vi "PVCamApp.vi"() -> ()   [LabVIEW 2018]
uses:
  D:/SVN/PM/sdk/AppSamples/LabVIEWSamples/trunk/Release/2018/Dependencies/PVCamNET.dll
  Dependencies/PVCamNET.dll
  SubVis/PVCamGlobalVariables.vi
panel:
  out "Name":string
  in  "Bayer pattern":string(combo)
  in  "Camera Control":enum32{"Basic", "Advanced", "Disk streaming"}(tab)
  out "Disk queue size":dbl
  out "Buffer Index":dbl
  in  "Scrollbar":i32(c297)
  in  "Exposure Time":dbl
  in  "Binning":string(combo)
  in  "X":u16
  in  "Width":u16
  in  "Y":u16
  in  "Height":u16
  in  "Full CCD":bool
  in  "Single Capture":bool
  in  "Live start":bool
  in  "Live stop":bool
  in  "Live status":bool
  in  "Get ROI":bool
  in  "Save Image to TIFF":bool
  out "Capturing":bool
  in  "Exposure Resolution":string(combo)
  out "8 Bit Histogram":i32[](graph)
  in  "Histogram On/Off":bool
  out "?":string
  out "Image saving path":string
  in  "Color (Off/On)":bool
  in  "Post-processing function value":dbl
  in  "Post-processing function":string(combo)
  in  "Readout ports and speeds":string(combo)
  in  "Gain":string(combo)
  in  "Sensor clearing mode":string(combo)
  in  "Clear Cycles":dbl
  in  "Trigger Out Behavior":string(combo)
  in  "Trigger In Behavior":string(combo)
  out "Stream Saving":bool
  in  "Disk streaming On/Off":bool
  in  "Format (0 for RAW[mono only] and 1 for TIFF[mono/color])":u8 max=1 step=1
  out "Disk stream saving path":string
  in  "Image saving path":path
  out "LabVIEW app version":string
  out "PVCamNET version":string
  out "Trigger Mode":i32
  out "Exposure":u32
  out "YBinning":u16
  out "XBinning":u16
  out "CC Min":u32
  out "CC Max":u32
  out "Exp. out":i32
  out "Clearing modes":i32
  out "Full CCD Y":i32
  out "Full CCD Height":i32
  out "Full CCD Width":i32
  out "Full CCD X":i32
  out "Y Binning":u32
  out "X Binning":u32
  in  "Init":bool
  in  "Camera status":bool
  in  "Close Camera":bool
  in  "Open Camera":bool
  in  "Select Camera":string(combo)
  in  "Uninit":bool
  in  "PVCam indicator":bool
  out "PVCam version":string
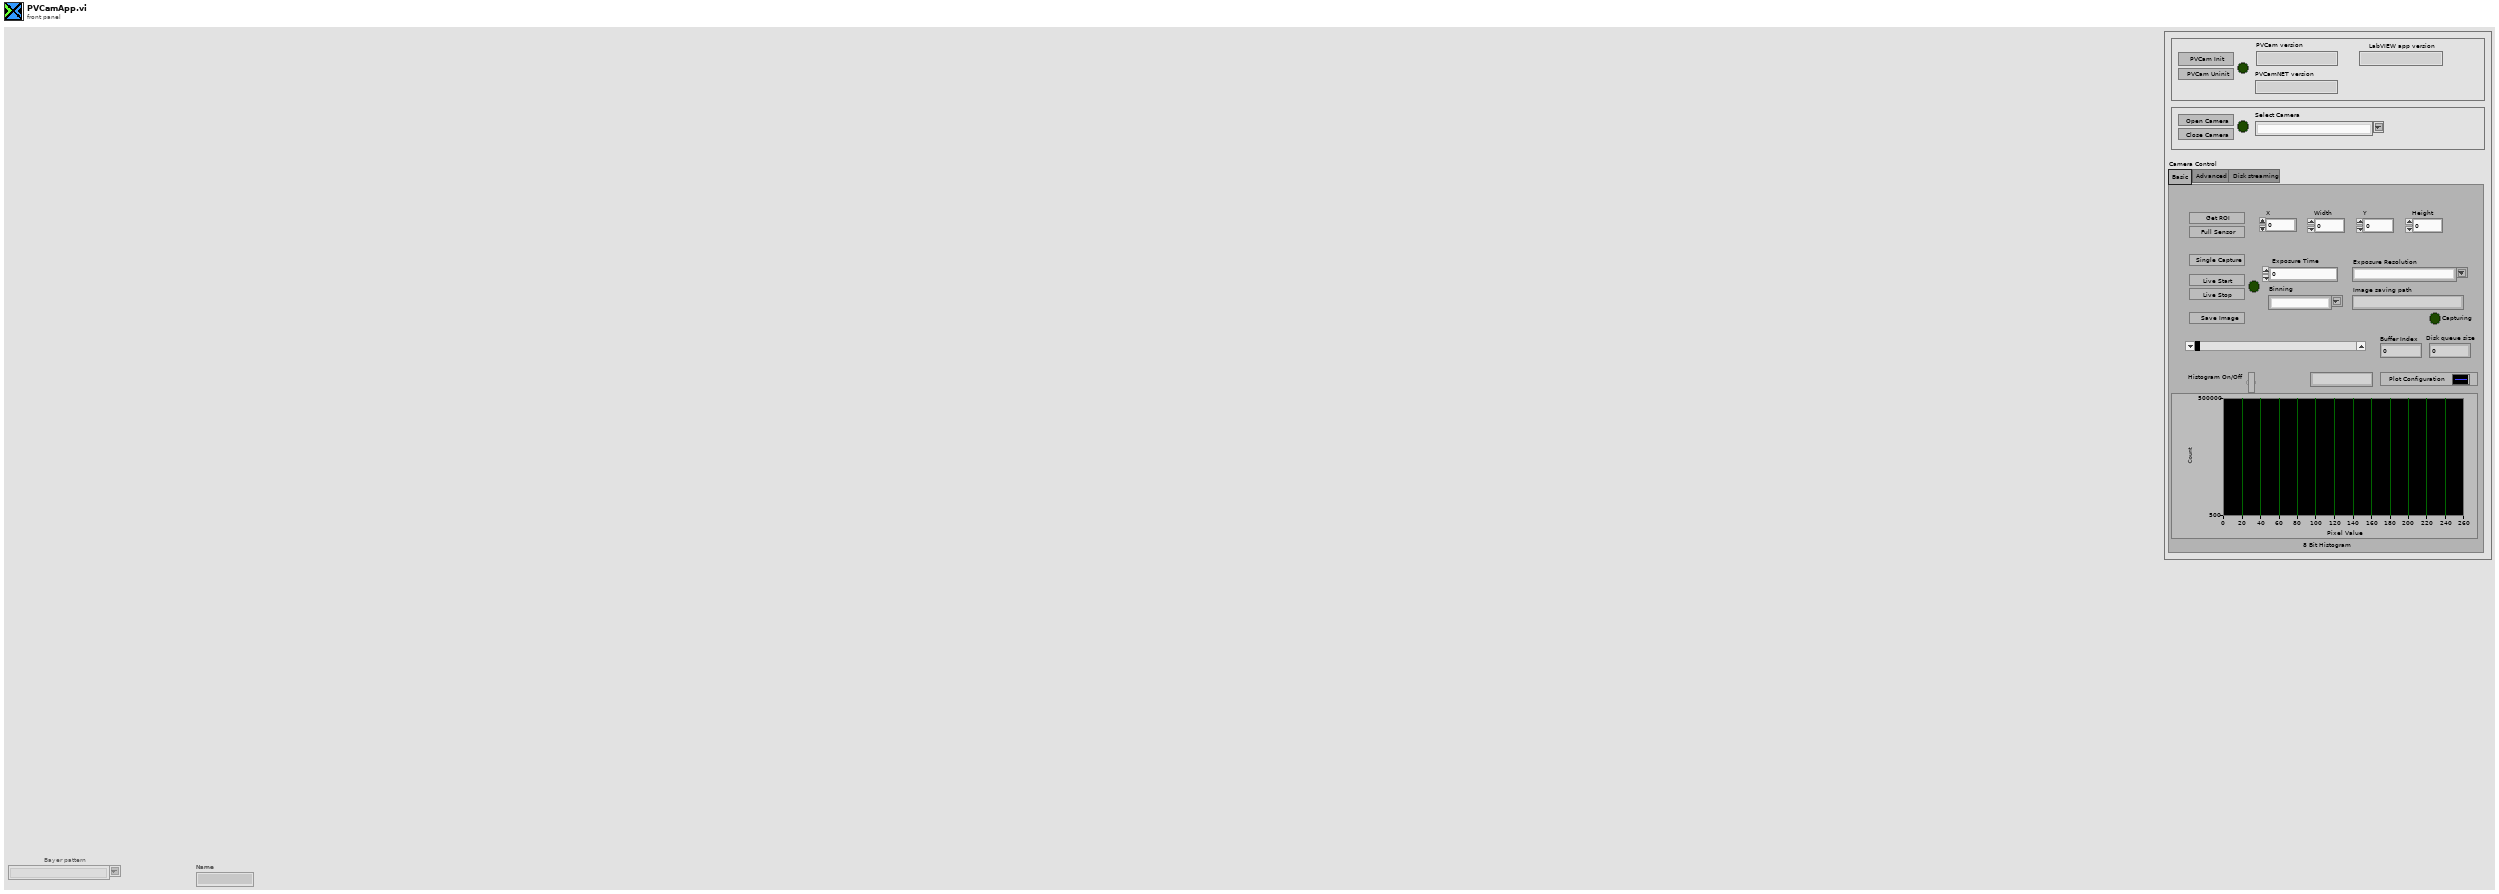
[diagram p1: front panel]
types:
  T1 = cluster{"Buffer Index":refnum<vi>, "Disk queue size":refnum<vi>, "Scrollbar":refnum<vi>}
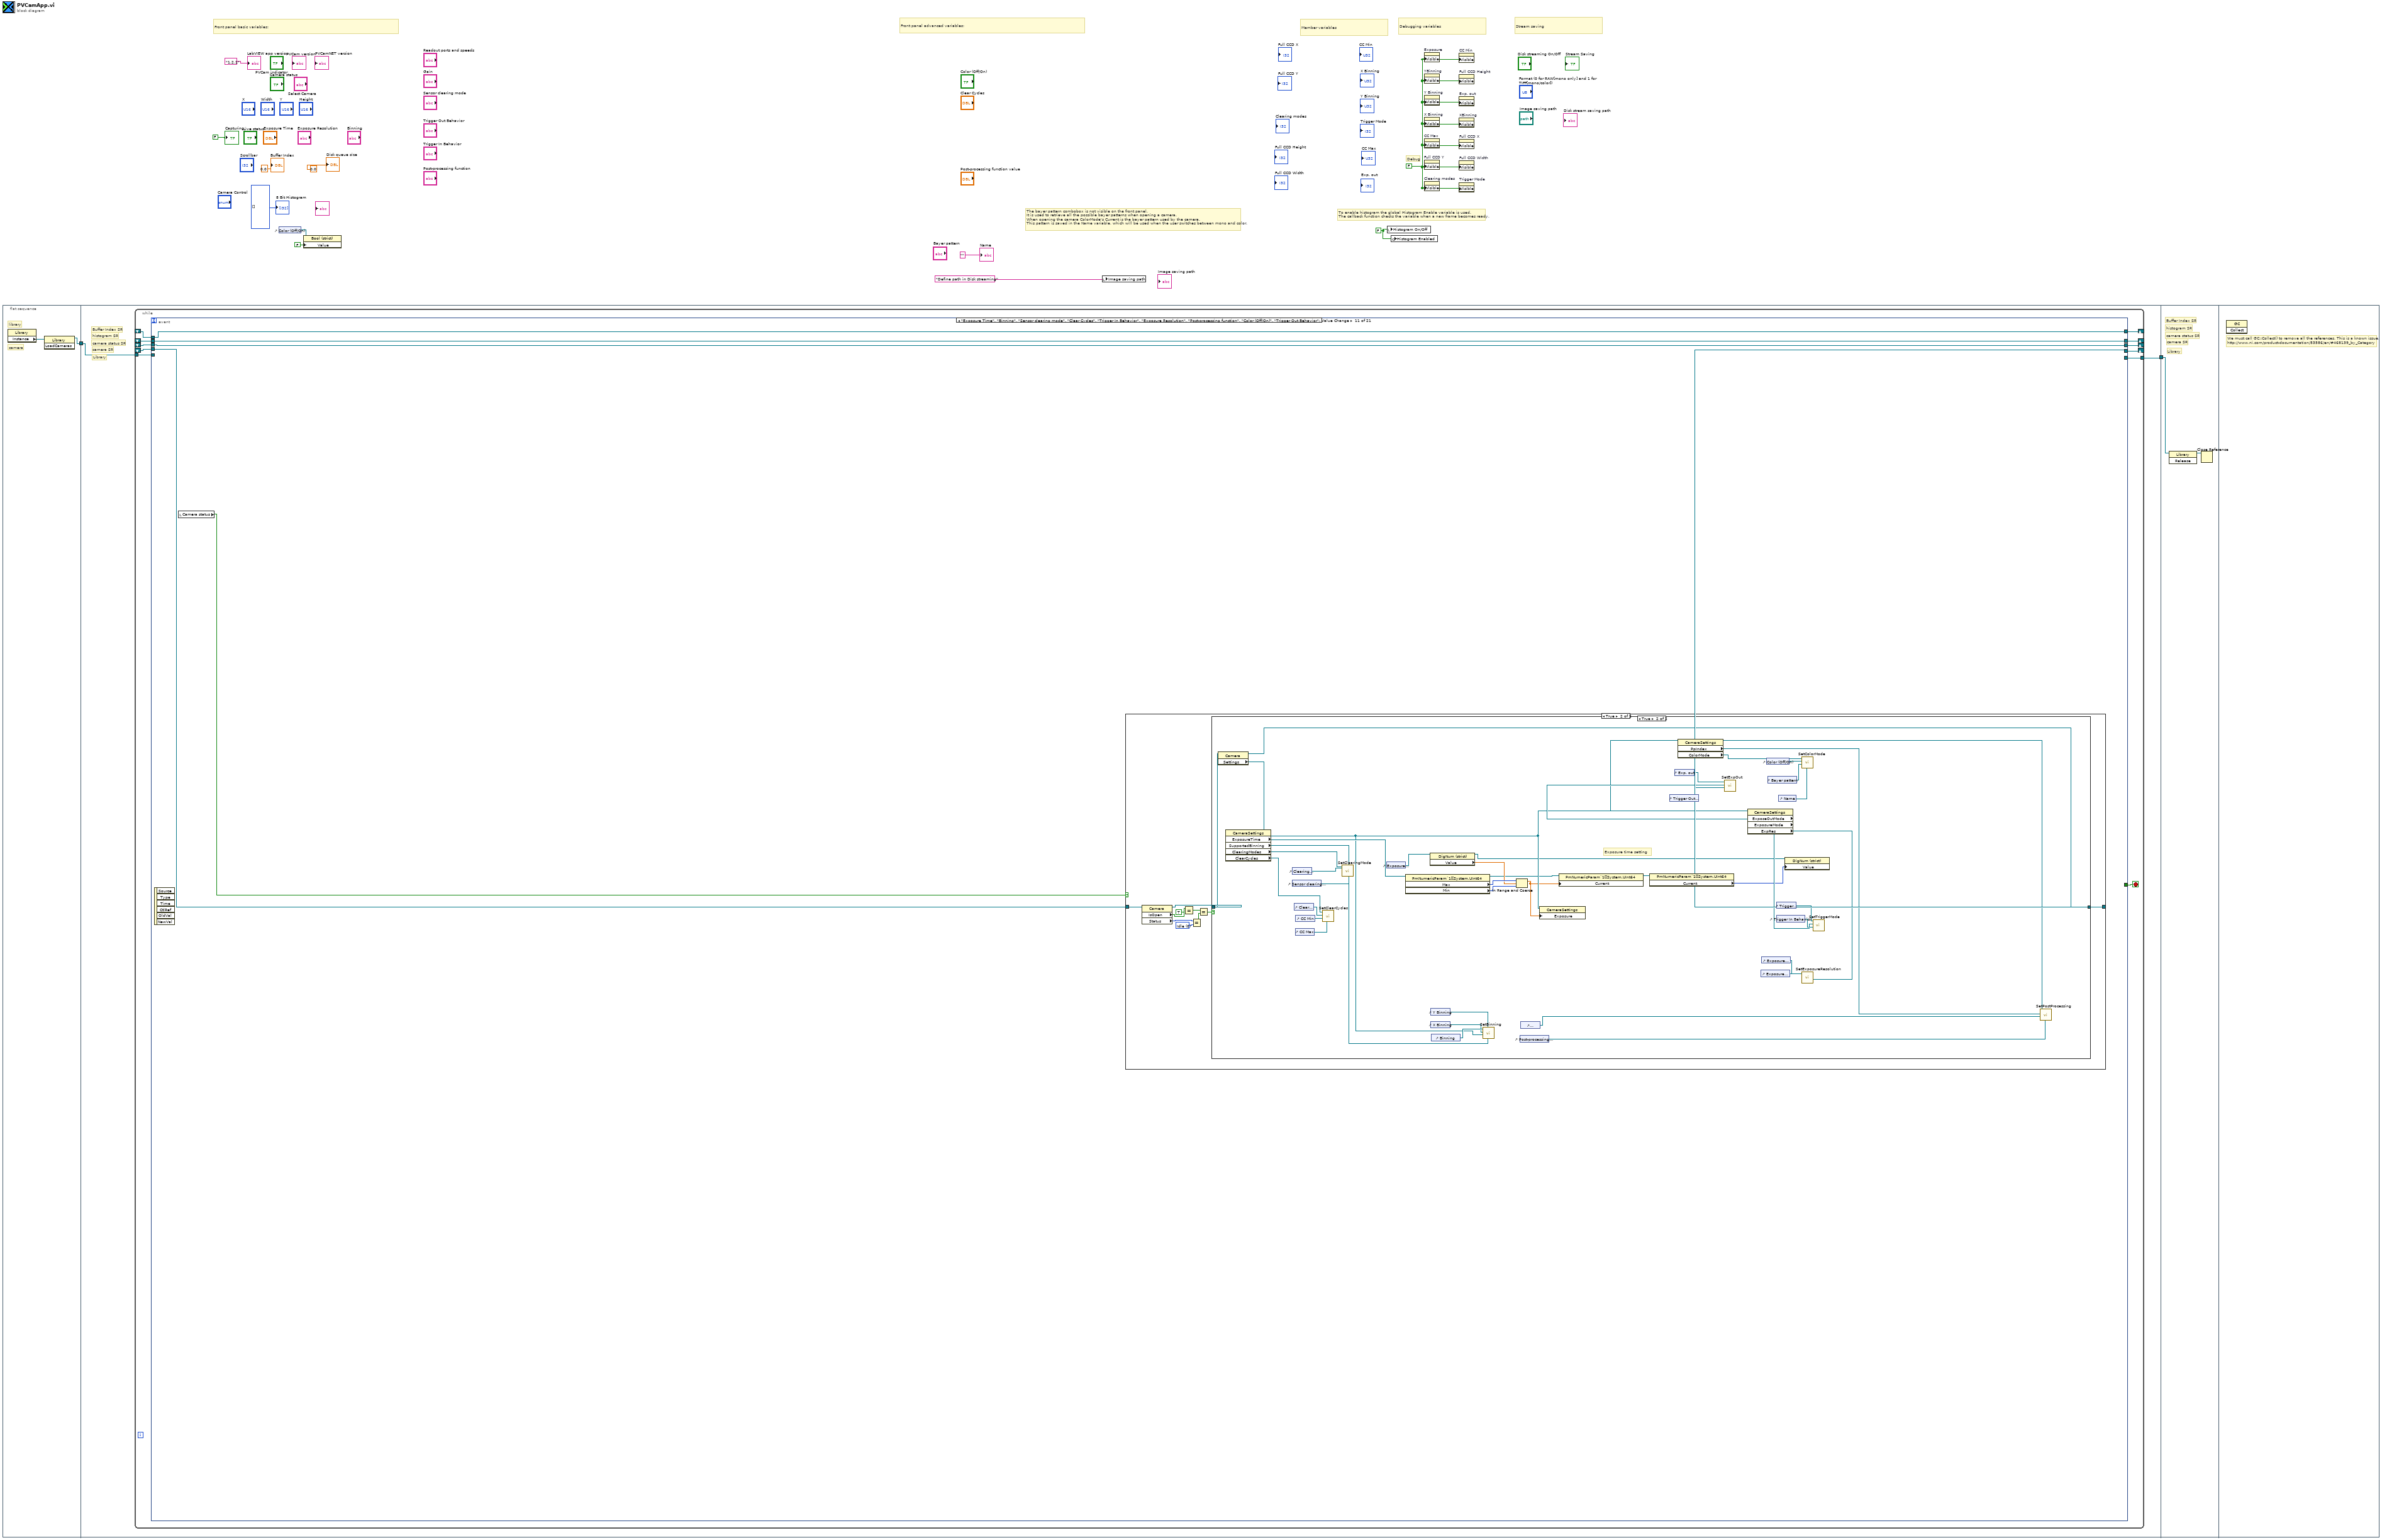
[diagram p0: block diagram]
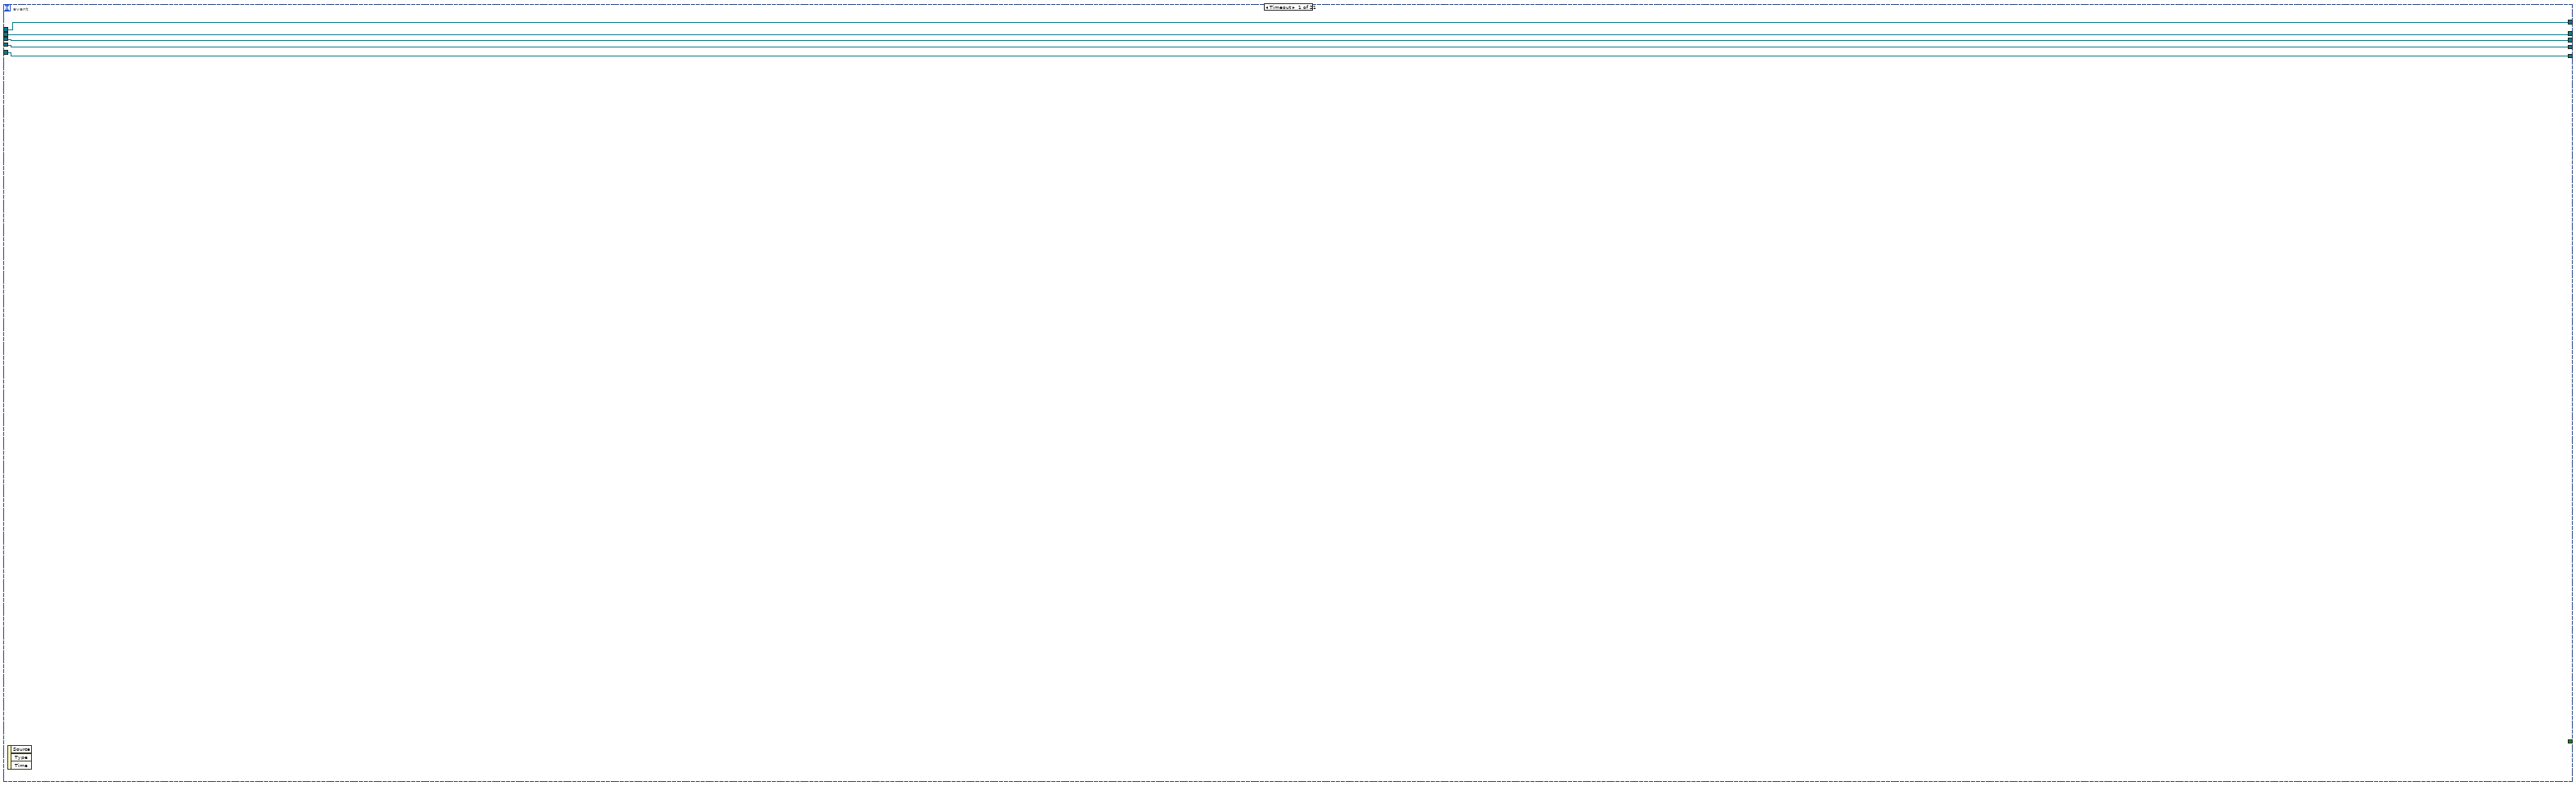
[diagram p2: hidden frame]
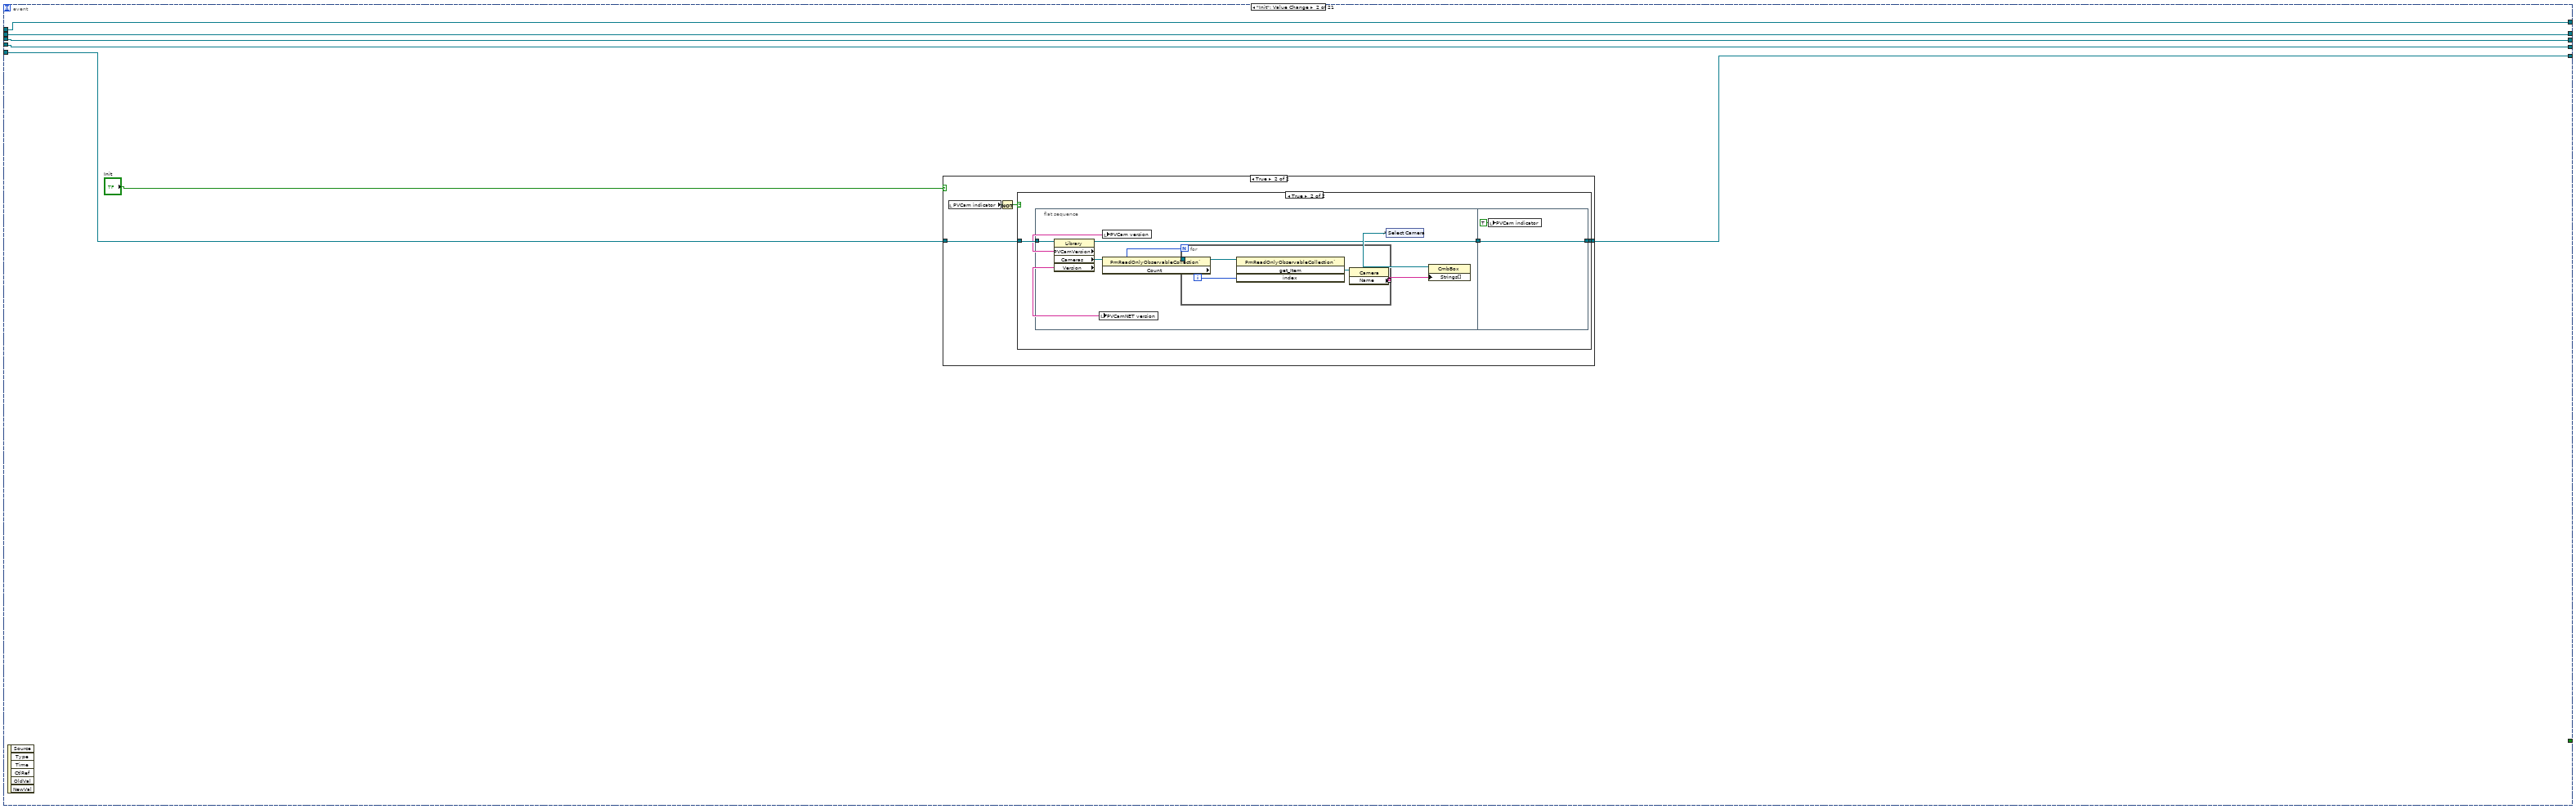
[diagram p3: hidden frame]
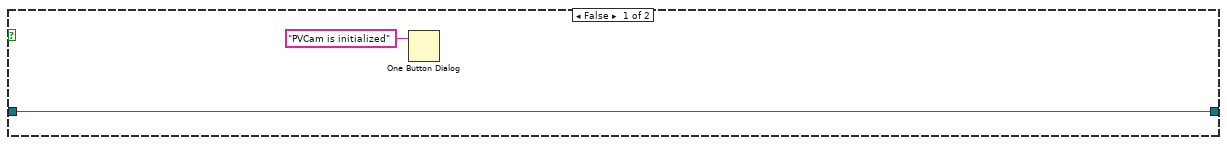
[diagram p5: hidden frame]
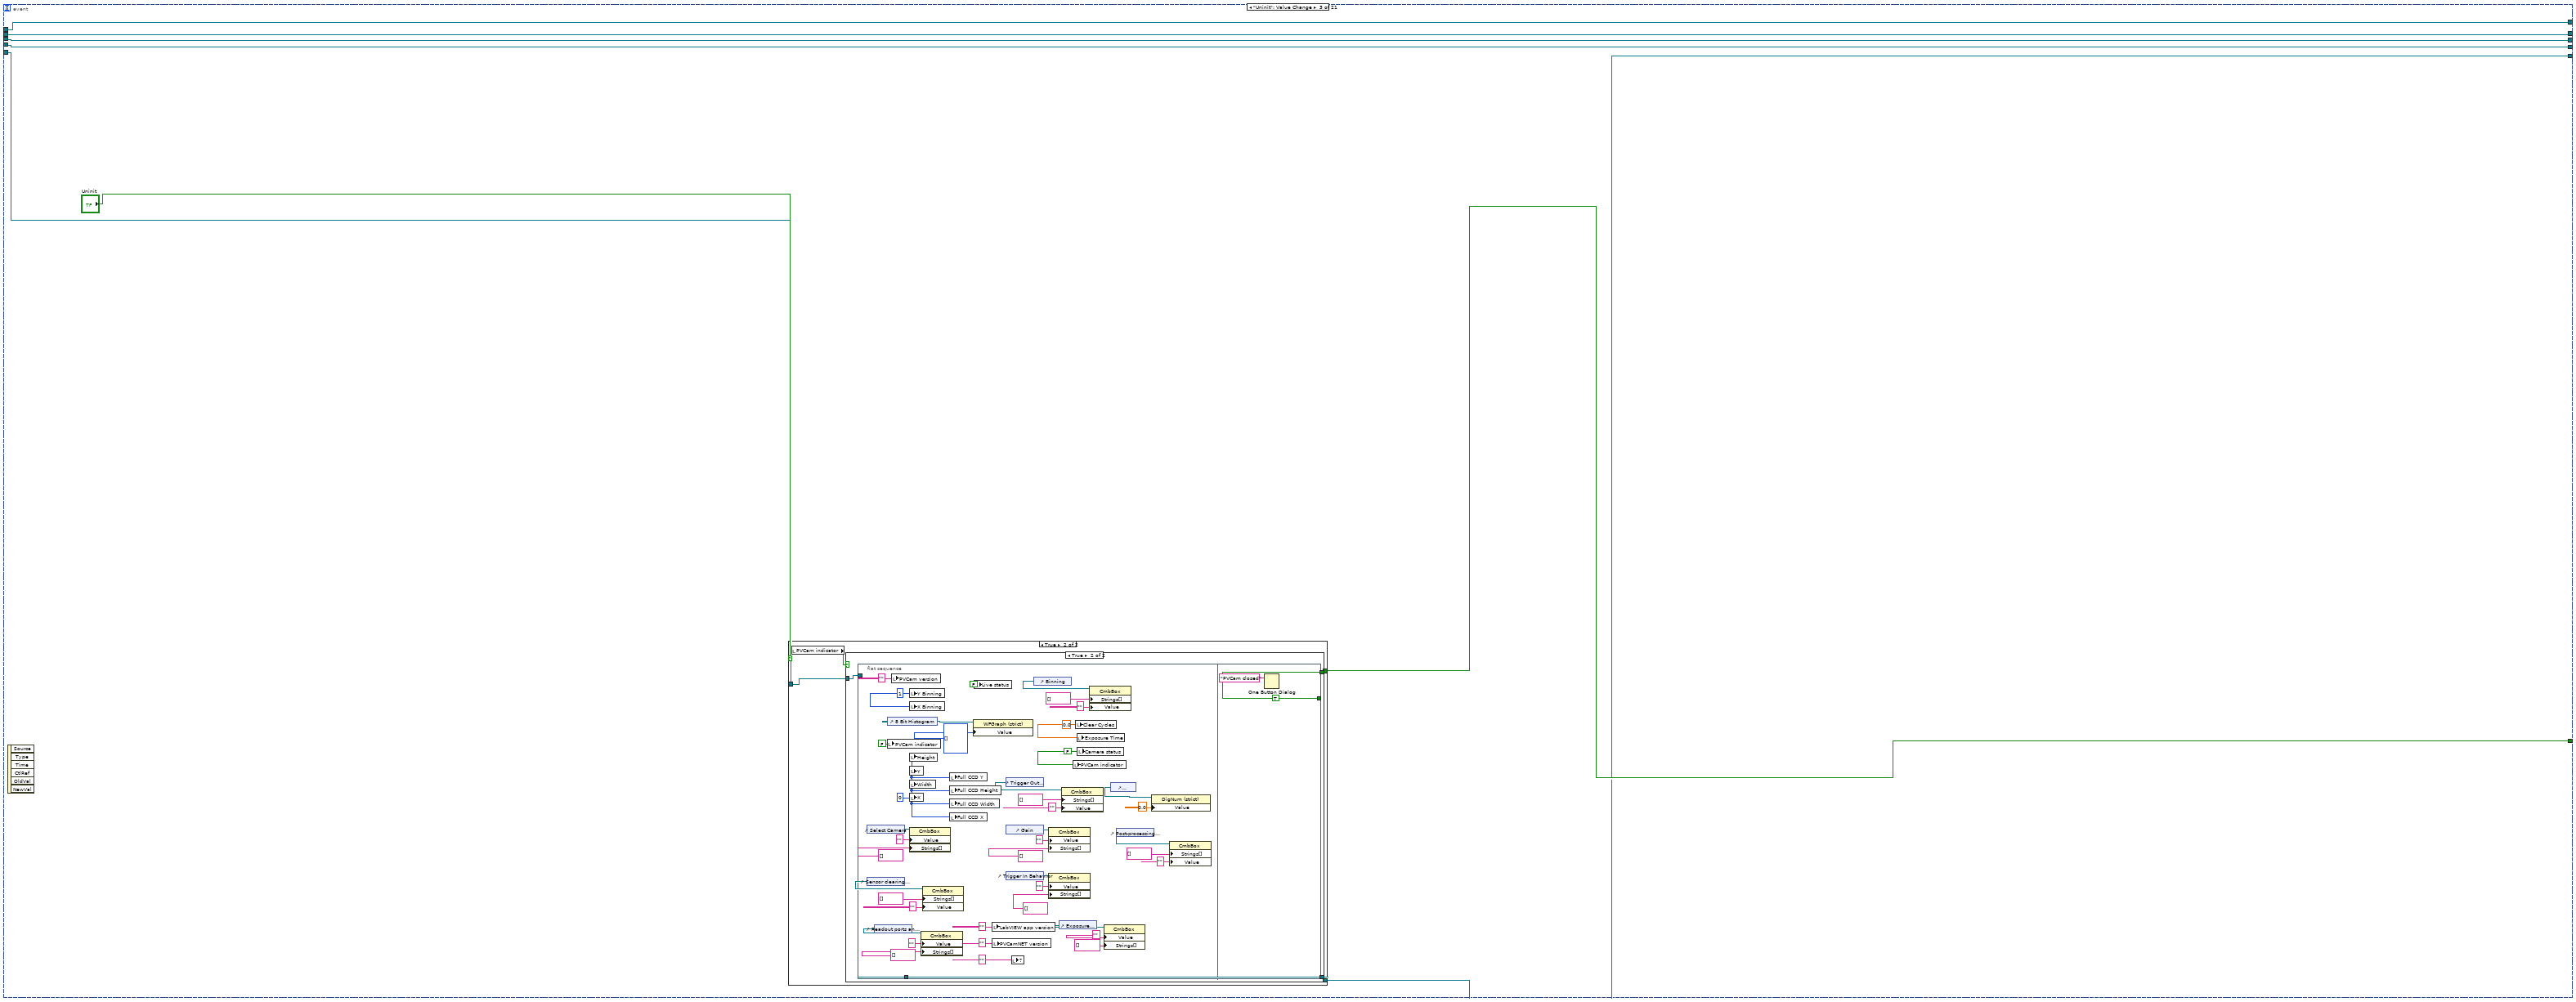
[diagram p6: hidden frame]
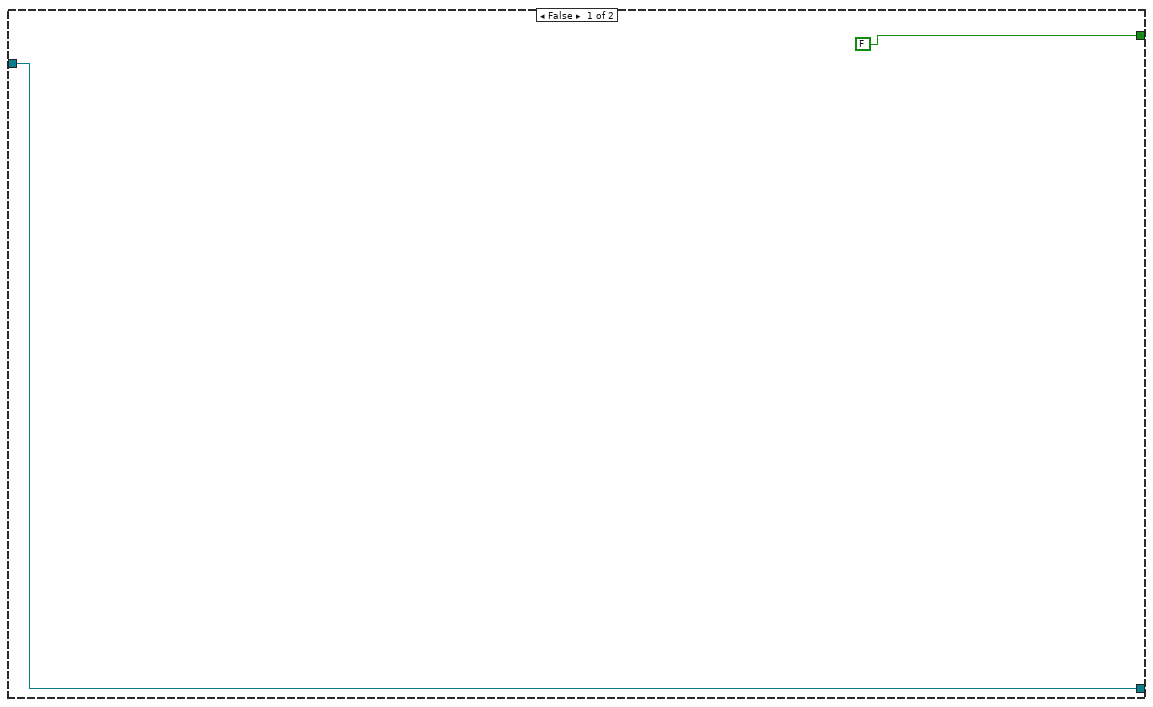
[diagram p7: hidden frame]
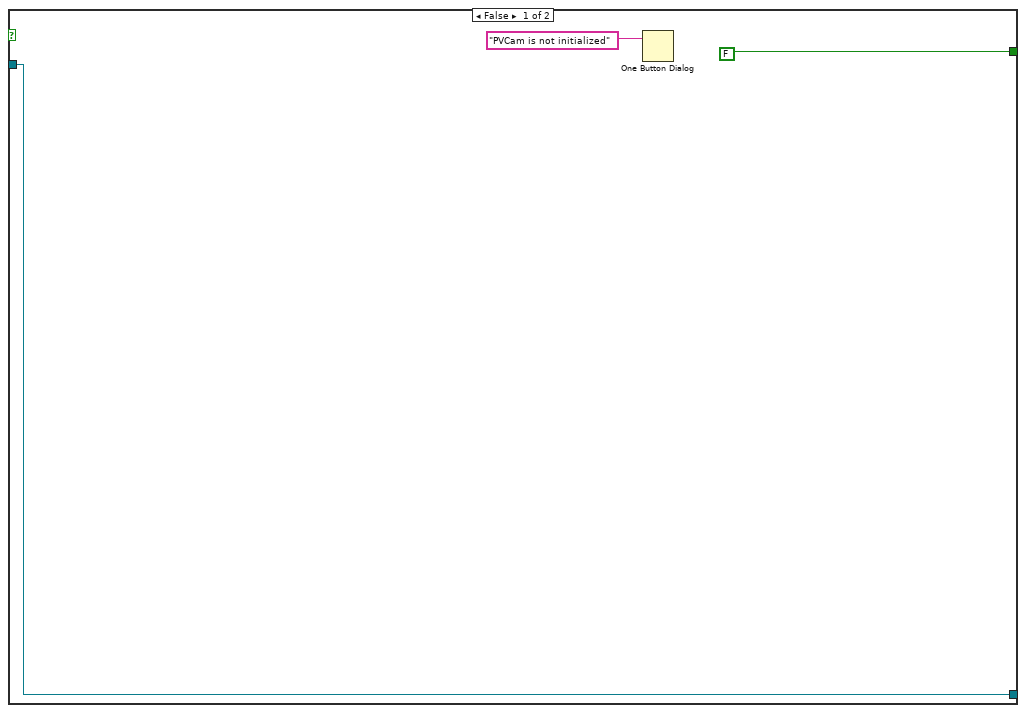
[diagram p8: hidden frame]
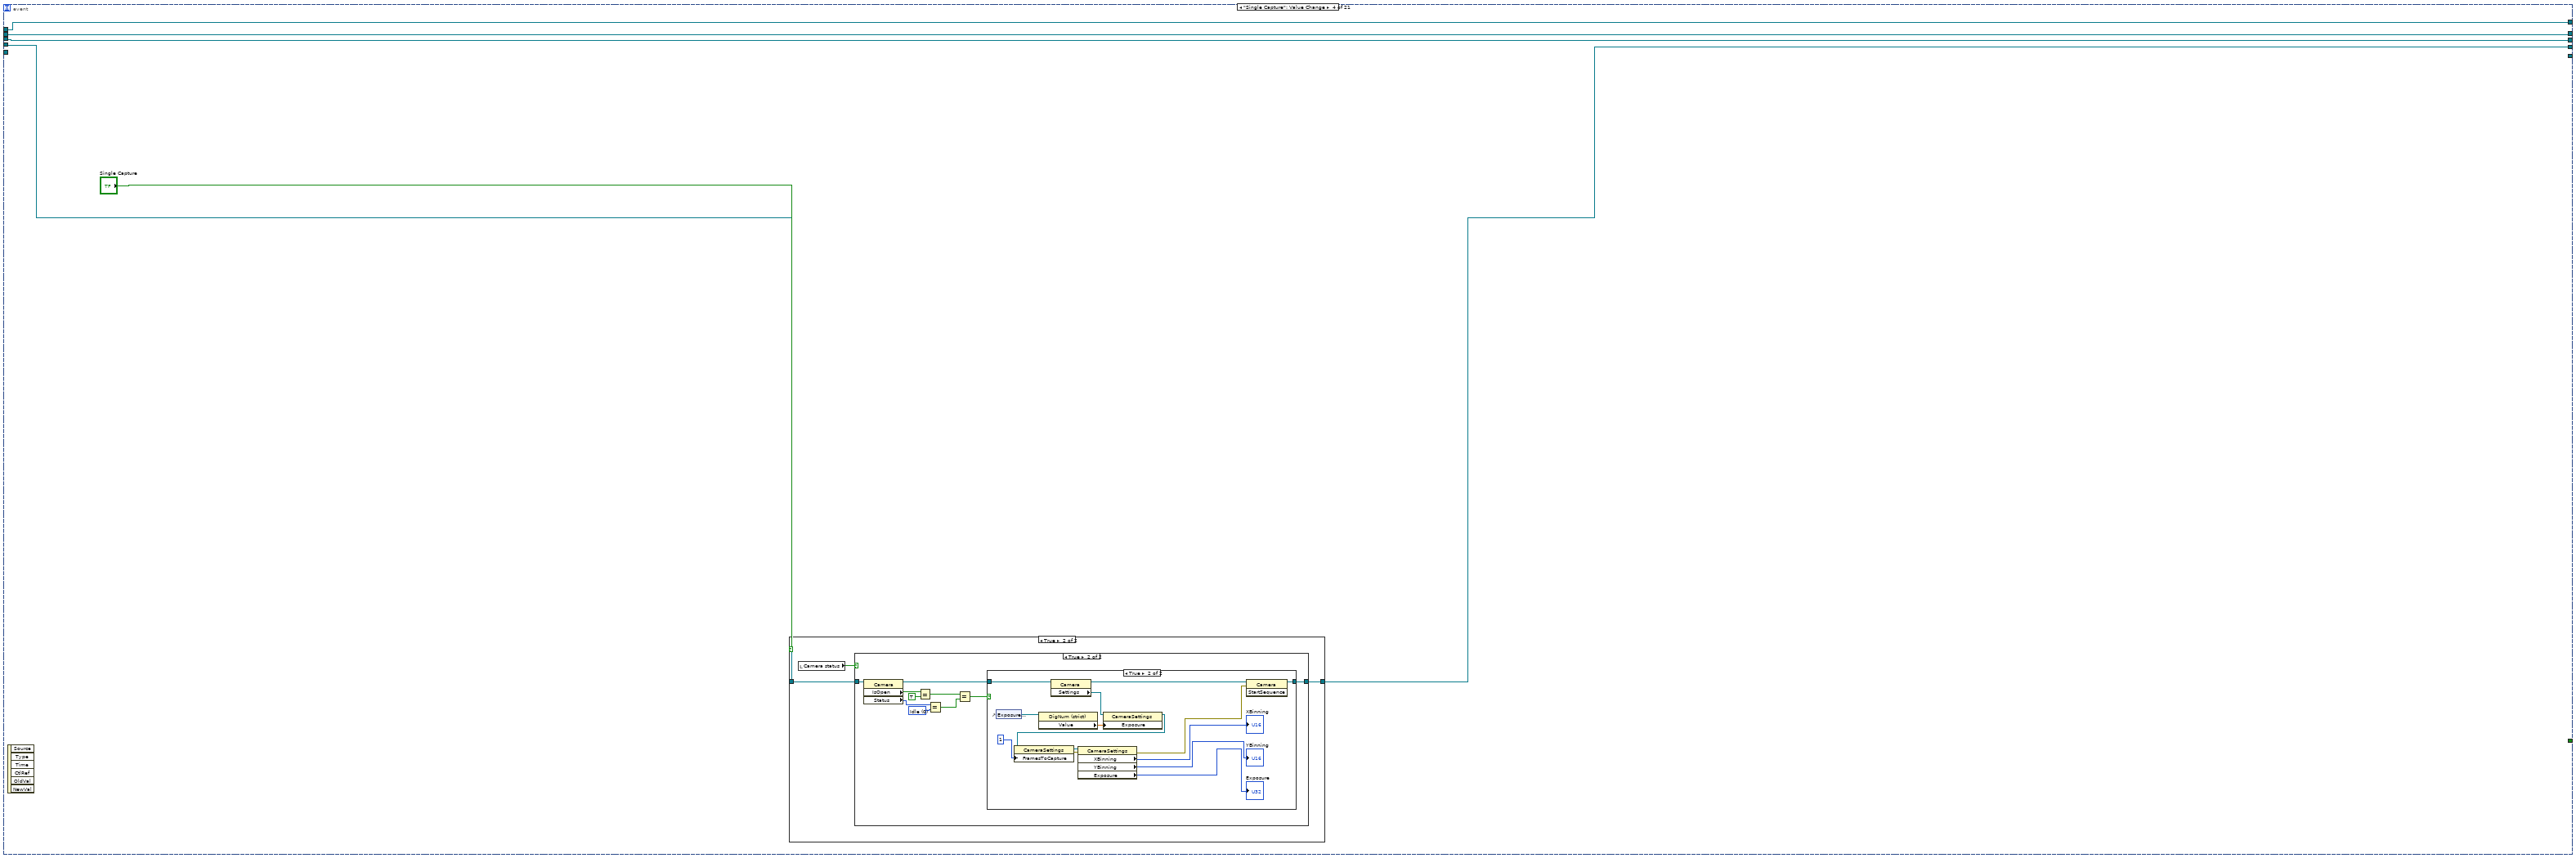
[diagram p9: hidden frame]
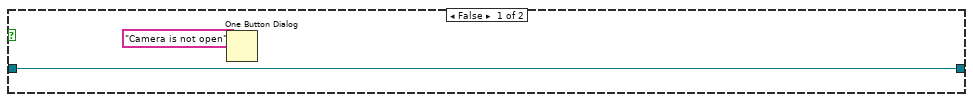
[diagram p11: hidden frame]
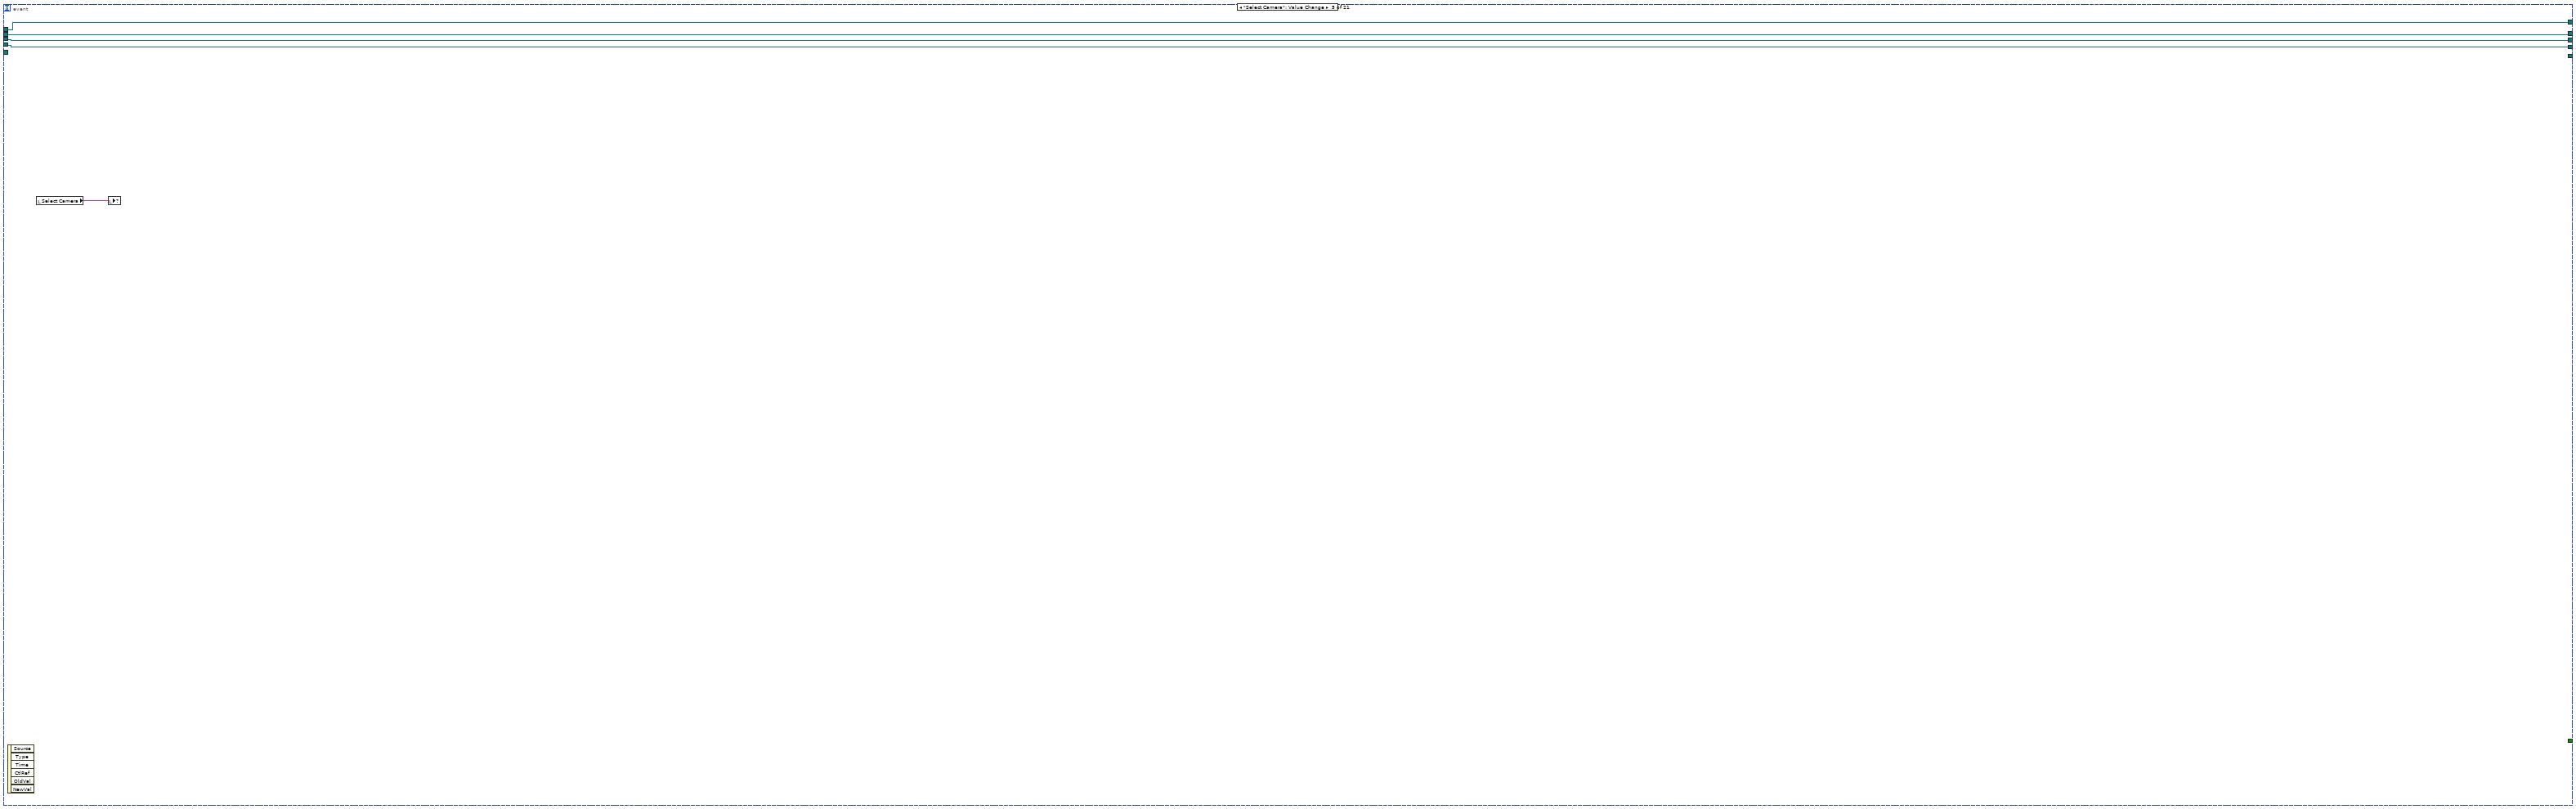
[diagram p13: hidden frame]
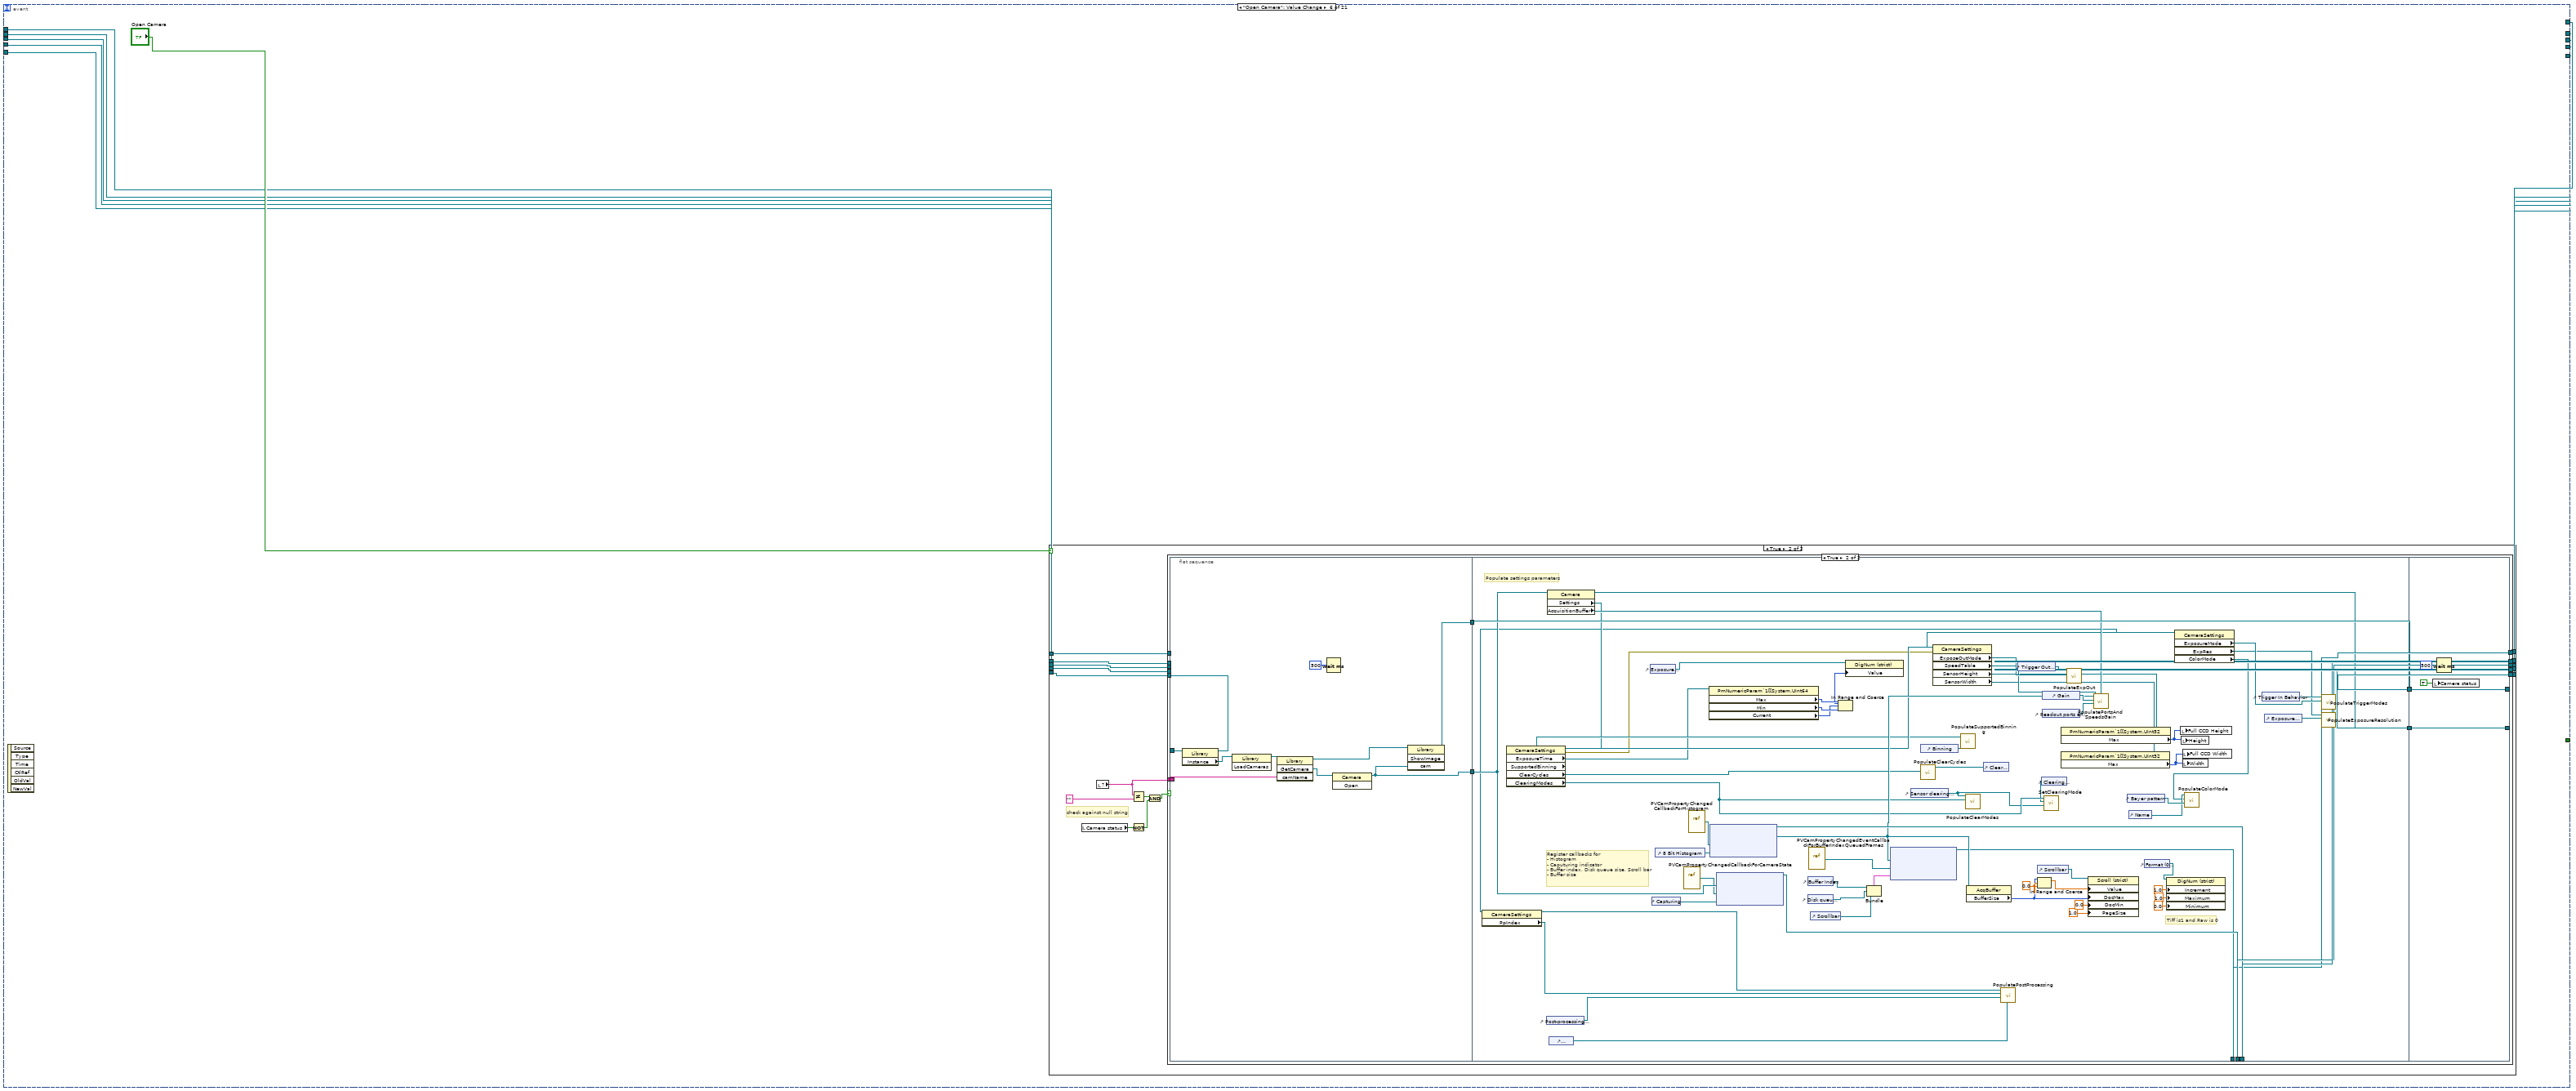
[diagram p14: hidden frame]
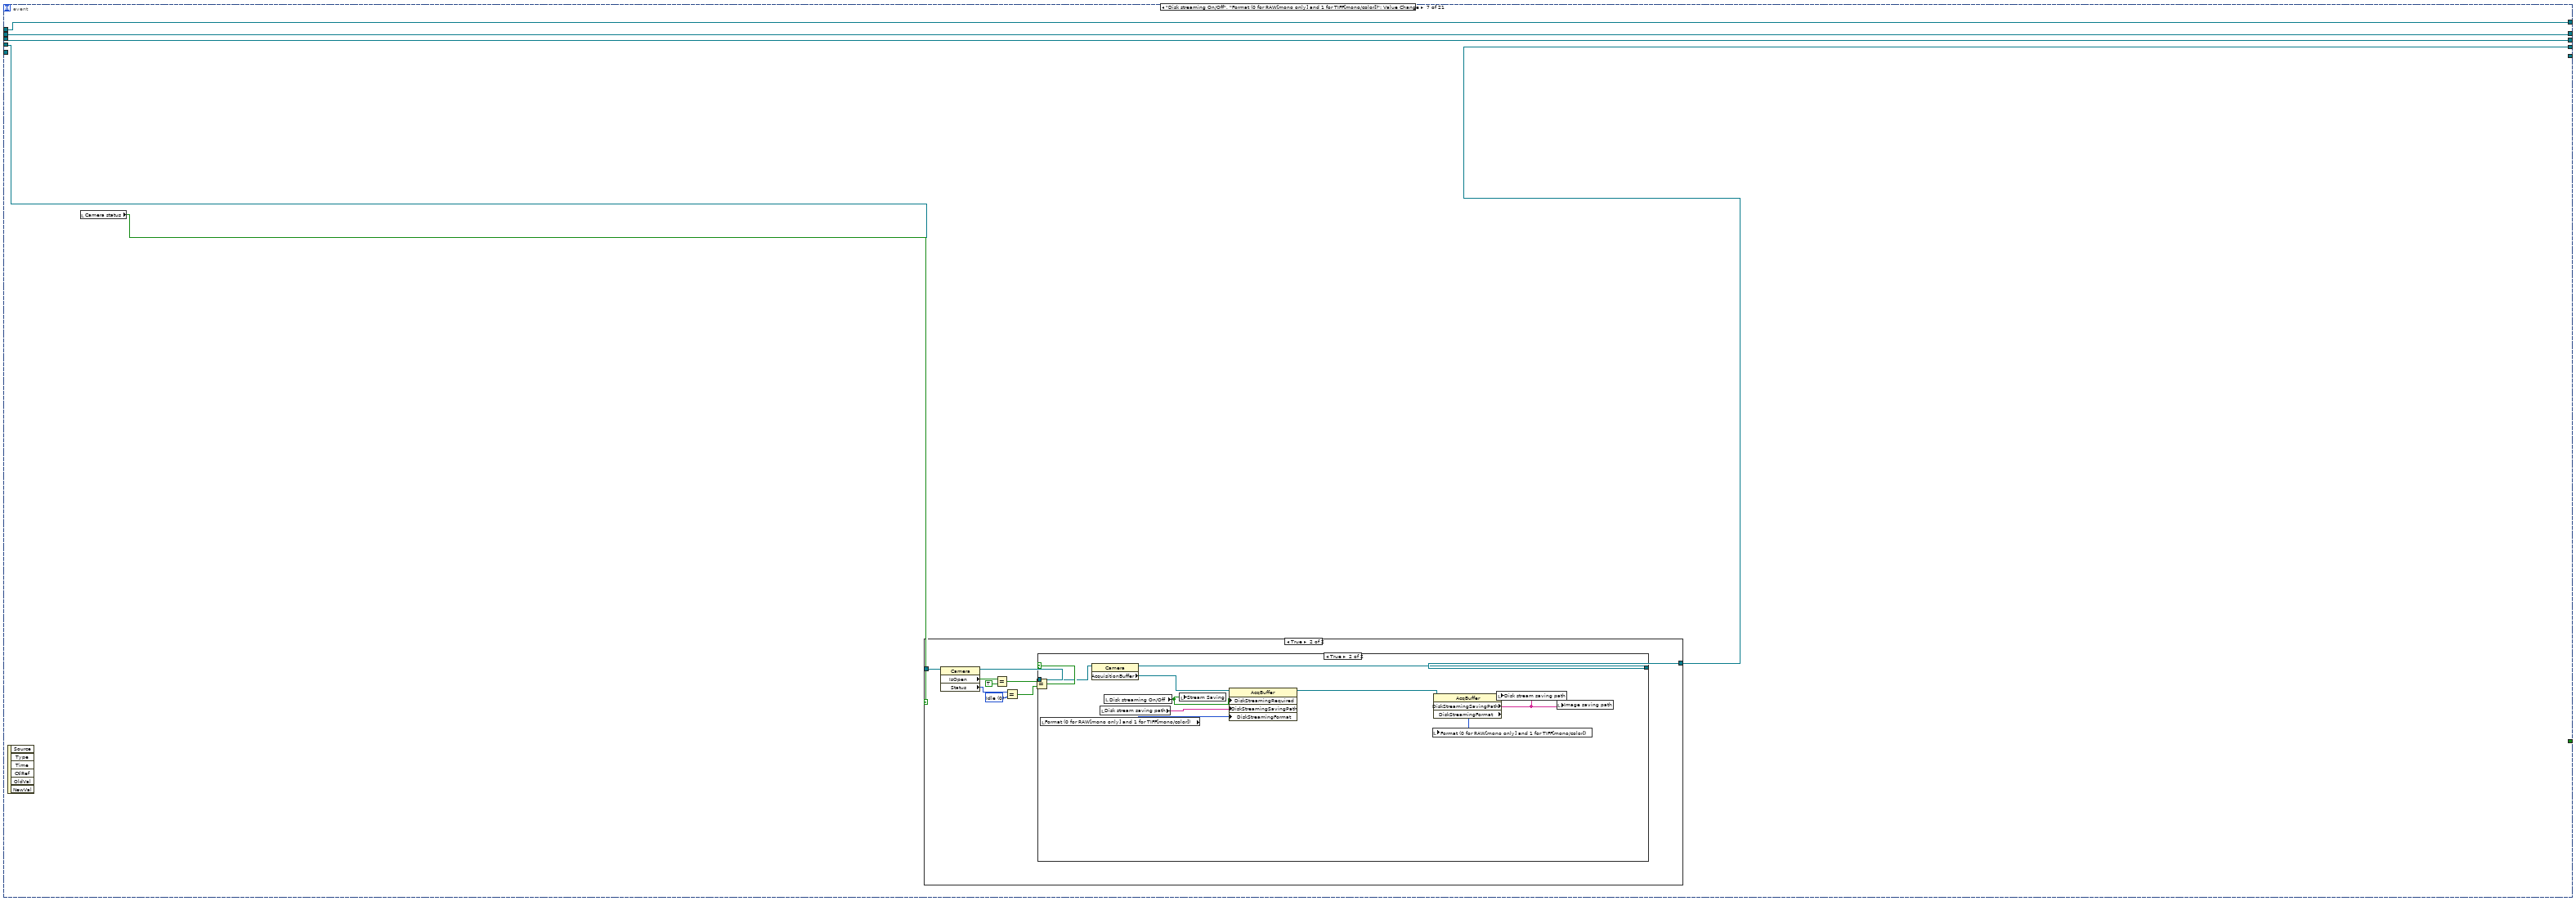
[diagram p17: hidden frame]
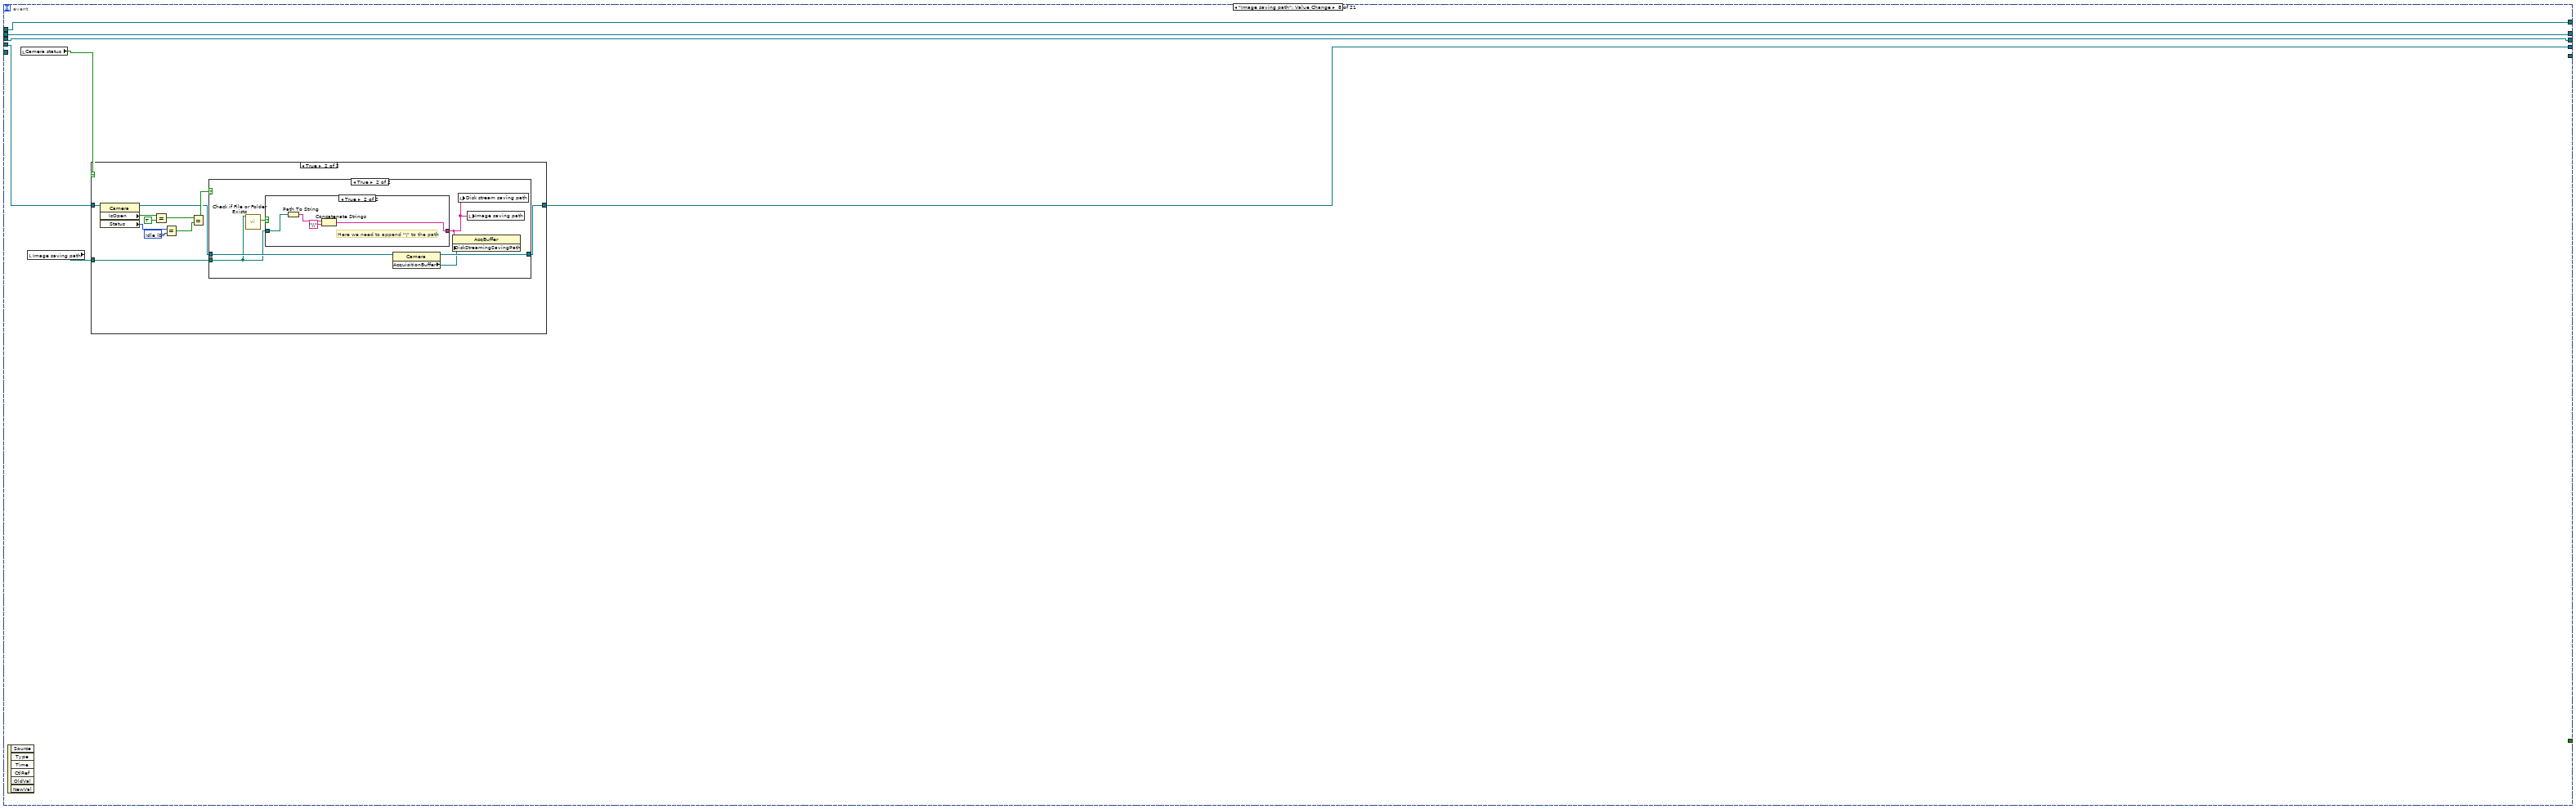
[diagram p20: hidden frame]
diagram:
  w7 = FALSE ("Histogram On/Off")
  w11 = FALSE ("Visible")
  # "Stream saving"
  # "To enable histogram the global Histogram Enable variable is used. \nThe callback function checks the variable when a new frame becomes ready."
  # "Debugging variables"
  # "Member variables"
  # "Front panel advanced variables:"
  # "Front panel basic variables:"
  # "The bayer pattern combobox is not visible on the front panel.\nIt is used to retrieve all the possible bayer patterns when opening a camera.\nWhen opening the camera ColorMode's Current is the bayer pattern used by the camera.\nThis pattern is saved in the Name variable, which will be used when the user switches between mono and color."
  # "Debug"
  n1 = flat-sequence {
    tunnel: [w15] -> w13
    tunnel: w13 -> [w16]
    tunnel: [w17] -> w12
    tunnel: w12 -> [w931]
    frame #0 {
      # "camera"
      # "library"
      n2 = property class="Library"() -> ("Instance"=w14:refnum<k24>)  [unwired: 2 in, 2 out]
      n3 = invoke class="Library" method="LoadCameras"(reference=w14) -> (reference out=w15:refnum<k24>)  [unwired: 2 in, 2 out]
    }
    frame #1 {
      # "Library"
      # "camera SR"
      # "Buffer Index SR"
      # "camera status SR"
      # "histogram SR"
      n4 = while {
        shift-right: [w24] -> _
        shift-left: _ -> [w25]
        tunnel: w16 -> [w27]
        tunnel: [w28] -> w17
        shift-right: [w23] -> _
        shift-left: _ -> [w22]
        shift-right: [w20] -> _
        shift-left: _ -> [w21]
        shift-right: [w18] -> _
        shift-left: _ -> [w19]
        stop <- w26 stop-if-true
        n5 = event shown="[10] \"Exposure Time\", \"Binning\", \"Sensor clearing mode\", \"Clear Cycles\", \"Trigger In Behavior\", \"Exposure Resolution\", \"Post-processing function\", \"Color (Off/On)\", \"Trigger Out Behavior\": Value Change" {
          selector: _ -> [_ _ _ _ _ _ _ _ _ _ _ _ _ _ _ _ _ _ _ _ _]
          dyn-events: _ -> [_ _ _ _ _ _ _ _ _ _ _ _ _ _ _ _ _ _ _ _ _]
          timeout: _ -> [_ _ _ _ _ _ _ _ _ _ _ _ _ _ _ _ _ _ _ _ _]
          tunnel: [w33 w40 w71 _ _ w179 _ _ _ _ _ _ _ _ _ _ _ _ _ _ _] -> w28
          tunnel: w27 -> [w33 w39 w70 _ _ w181 _ _ _ _ _ _ _ _ _ _ _ _ _ _ _]
          tunnel: [_ _ w72 _ _ _ _ _ _ _ _ _ _ _ _ _ _ _ _ _ _] -> w26
          tunnel: w25 -> [w32 w37 w69 w130 w169 w180 w301 w330 w363 w488 w526 w589 w614 w653 w680 w702 w738 w818 w859 w890 w915]
          tunnel: [w32 w37 w69 w134 w169 w178 w300 w324 w364 w484 w528 w585 w613 w652 w679 w701 w734 w817 w858 w889 w914] -> w24
          tunnel: [w31 w36 w67 w133 w170 w177 w298 w326 w361 w487 w525 w587 w612 w650 w678 w699 w736 w815 w857 w888 w918] -> w23
          tunnel: w22 -> [w31 w36 w67 w133 w170 w176 w298 w326 w362 w487 w525 w587 w612 w650 w678 w699 w736 w815 w857 w888 w918]
          tunnel: [w30 w34 w68 w132 w168 w175 w297 w325 w357 w486 w524 w586 w611 w649 w677 w698 w735 w814 w856 w887 w917] -> w20
          tunnel: w21 -> [w30 w34 w68 w132 w168 w174 w297 w325 w360 w486 w524 w586 w611 w649 w677 w698 w735 w814 w856 w887 w917]
          tunnel: w19 -> [w29 w35 w66 w131 w167 w173 w299 w327 w359 w485 w523 w588 w610 w651 w676 w700 w733 w813 w855 w886 w916]
          tunnel: [w29 w35 w66 w131 w167 w172 w299 w327 w358 w485 w523 w588 w610 w651 w676 w700 w733 w813 w855 w886 w916] -> w18
          event Timeout {
            n6 = event-data() -> ()  [unwired: 1 in, 3 out]
          }
          event "Init": Value Change {
            n7 = event-data() -> ()  [unwired: 1 in, 6 out]
            n8 = case shown="True" "Init" {
              tunnel: [w41 w44] -> w40
              tunnel: w39 -> [w41 w45]
              frame False {
              }
              frame True {
                n9 = local read "PVCam indicator"() -> (w43:bool)
                n10 = Not(x=w43) -> (.not. x?=w42:bool)
                n11 = case shown="True" w42 {
                  tunnel: w45 -> [w47 w49]
                  tunnel: [w47 w48] -> w44
                  frame False {
                    n12 = One Button Dialog(message="PVCam is initialized") -> ()  [unwired: 1 in, 1 out]
                  }
                  frame True {
                    n13 = flat-sequence {
                      tunnel: w49 -> [w59]
                      tunnel: [w52] -> w50
                      tunnel: [w65] -> w48
                      tunnel: w50 -> [w65]
                      frame #0 {
                        n14 = property class="Library"(reference=w59) -> (reference out=w52:refnum<k24>, "PVCamVersion"=w58:string, "Cameras"=w57:refnum<k24>, "Version"=w51:string)  [unwired: 1 in, 1 out]
                        n15 = local write "PVCamNET version"(w51) -> ()
                        n16 = local write "PVCam version"(w58) -> ()
                        n17 = property class="PmReadOnlyObservableCollection`"(reference=w57) -> (reference out=w55:refnum<k24>, "Count"=w56:i32)  [unwired: 1 in, 1 out]
                        n18 = for {
                          N: w56 -> [_]
                          tunnel: w55 -> [w63]
                          tunnel: [w60] -> w53 mode=indexing
                          i -> [w62]
                          n19 = invoke class="PmReadOnlyObservableCollection`" method="get_Item"(reference=w63, "index"=w62) -> ("get_Item"=w61:refnum<k24>)  [unwired: 2 in, 3 out]
                          n20 = property class="Camera"(reference=w61) -> ("Name"=w60:string)  [unwired: 1 in, 2 out]
                        }
                        n21 = control-ref of="Select Camera"() -> (w54:refnum<vi>)
                        n22 = property class="CmbBox"(reference=w54, "Strings[]"=w53) -> ()  [unwired: 1 in, 2 out]
                      }
                      frame #1 {
                        n23 = local write "PVCam indicator"(TRUE ("PVCam status")) -> ()
                      }
                    }
                  }
                }
              }
            }
          }
          event "Uninit": Value Change {
            n24 = event-data() -> ()  [unwired: 1 in, 6 out]
            n25 = case shown="True" "Uninit" {
              tunnel: [FALSE ("PVCam status") w79] -> w72
              tunnel: [w74 w78] -> w71
              tunnel: w70 -> [w74 w77]
              frame False {
              }
              frame True {
                n26 = local read "PVCam indicator"() -> (w76:bool)
                n27 = case shown="True" w76 {
                  tunnel: [FALSE ("PVCam status") w85] -> w79
                  tunnel: [w82 w83] -> w78
                  tunnel: w77 -> [w82 w84]
                  frame False {
                    n28 = One Button Dialog(message="PVCam is not initialized") -> ()  [unwired: 1 in, 1 out]
                  }
                  frame True {
                    n29 = flat-sequence {
                      tunnel: [w121] -> w83
                      tunnel: w84 -> [w121]
                      tunnel: [TRUE ("PVCam status")] -> w85
                      frame #0 {
                        w111 = u32 1 ("Y Binning")
                        w110 = 0.0 ("Clear Cycle")
                        w109 = FALSE ("Camera Status")
                        w108 = 0 ("Full CCD Y")
                        n30 = control-ref of="Select Camera"() -> (w125:refnum<vi>)
                        n31 = control-ref of="Sensor clearing mode"() -> (w119:refnum<vi>)
                        n32 = control-ref of="Readout ports and speeds"() -> (w102:refnum<vi>)
                        n33 = local write "PVCam indicator"(FALSE ("PVCam status")) -> ()
                        n34 = control-ref of="8 Bit Histogram"() -> (w95:refnum<vi>)
                        n35 = local write "PVCam version"("" ("PVCam version")) -> ()
                        n36 = local write "Y Binning"(w111) -> ()
                        n37 = local write "X Binning"(w111) -> ()
                        n38 = local write "Height"(w108) -> ()
                        n39 = local write "Y"(w108) -> ()
                        n40 = local write "Width"(w108) -> ()
                        n41 = local write "X"(w108) -> ()
                        n42 = property class="CmbBox"(reference=w125, "Value"="", "Strings[]"=string[] [] ("Strings []")) -> ()  [unwired: 1 in, 2 out]
                        n43 = property class="CmbBox"(reference=w102, "Value"="", "Strings[]"=string[] [] ("Strings []")) -> ()  [unwired: 1 in, 2 out]
                        n44 = property class="CmbBox"(reference=w119, "Strings[]"=string[] [] ("Strings []"), "Value"="") -> ()  [unwired: 1 in, 2 out]
                        n45 = local write "Full CCD Y"(w108) -> ()
                        n46 = local write "Full CCD Height"(w108) -> ()
                        n47 = local write "Full CCD Width"(w108) -> ()
                        n48 = local write "Full CCD X"(w108) -> ()
                        n49 = property class="WFGraph (strict)"(reference=w95, "Value"=i32[] []) -> ()  [unwired: 1 in, 2 out]
                        n50 = local write "Live status"(FALSE ("Live")) -> ()
                        n51 = local write "LabVIEW app version"("" ("LabVIEW app version")) -> ()
                        n52 = local write "PVCamNET version"("" ("PVCamNET version")) -> ()
                        n53 = control-ref of="Trigger Out Behavior"() -> (w120:refnum<vi>)
                        n54 = control-ref of="Gain"() -> (w101:refnum<vi>)
                        n55 = control-ref of="Trigger In Behavior"() -> (w100:refnum<vi>)
                        n56 = local write item#7("" ("PVCam version")) -> ()
                        n57 = control-ref of="Binning"() -> (w118:refnum<vi>)
                        n58 = property class="CmbBox"(reference=w101, "Value"="", "Strings[]"=string[] [] ("Strings []")) -> ()  [unwired: 1 in, 2 out]
                        n59 = property class="CmbBox"(reference=w100, "Value"="", "Strings[]"=string[] [] ("Strings []")) -> ()  [unwired: 1 in, 2 out]
                        n60 = control-ref of="Exposure Resolution"() -> (w91:refnum<vi>)
                        n61 = property class="CmbBox"(reference=w120, "Strings[]"=string[] [] ("Strings []"), "Value"="") -> ()  [unwired: 1 in, 2 out]
                        n62 = local write "PVCam indicator"(w109) -> ()
                        n63 = local write "Clear Cycles"(w110) -> ()
                        n64 = local write "Exposure Time"(w110) -> ()
                        n65 = local write "Camera status"(w109) -> ()
                        n66 = property class="CmbBox"(reference=w118, "Strings[]"=string[] [] ("Strings []"), "Value"="") -> ()  [unwired: 1 in, 2 out]
                        n67 = property class="CmbBox"(reference=w91, "Value"="", "Strings[]"=string[] [] ("Strings []")) -> ()  [unwired: 1 in, 2 out]
                        n68 = control-ref of="Post-processing function value"() -> (w86:refnum<vi>)
                        n69 = control-ref of="Post-processing function"() -> (w87:refnum<vi>)
                        n70 = property class="DigNum (strict)"(reference=w86, "Value"=0.0) -> ()  [unwired: 1 in, 2 out]
                        n71 = property class="CmbBox"(reference=w87, "Strings[]"=string[] [] ("Strings []"), "Value"="") -> ()  [unwired: 1 in, 2 out]
                      }
                      frame #1 {
                        n72 = One Button Dialog(message="PVCam closed") -> ()  [unwired: 1 in, 1 out]
                      }
                    }
                  }
                }
              }
            }
          }
          event "Single Capture": Value Change {
            n73 = event-data() -> ()  [unwired: 1 in, 6 out]
            n74 = case shown="True" "Single Capture" {
              tunnel: w130 -> [w136 w138]
              tunnel: [w136 w139] -> w134
              frame False {
              }
              frame True {
                n75 = local read "Camera status"() -> (w137:bool)
                n76 = case shown="True" w137 {
                  tunnel: [w141 w151] -> w139
                  tunnel: w138 -> [w141 w150]
                  frame False {
                    n77 = One Button Dialog(message="Camera is not open") -> ()  [unwired: 1 in, 1 out]
                  }
                  frame True {
                    w148 = 0 items=["Idle", "Capturing"] ("Status")
                    n78 = property class="Camera"(reference=w150) -> (reference out=w142:refnum<k24>, "IsOpen"=w147:bool, "Status"=w149:i32)  [unwired: 1 in, 1 out]
                    n79 = Equal?(x=w147, y=TRUE) -> (x = y?=w145:bool)
                    n80 = Equal?(x=w149, y=w148) -> (x = y?=w144:bool)
                    n81 = Equal?(x=w145, y=w144) -> (x = y?=w143:bool)
                    n82 = case shown="True" w143 {
                      tunnel: [w152 w164] -> w151
                      tunnel: w142 -> [w152 w166]
                      frame False {
                      }
                      frame True {
                        n83 = control-ref of="Exposure Time"() -> (w162:refnum<vi>)
                        n84 = property class="DigNum (strict)"(reference=w162) -> ("Value"=w161:dbl)  [unwired: 1 in, 2 out]
                        n85 = property class="Camera"(reference=w166) -> (reference out=w165:refnum<k24>, "Settings"=w163:refnum<k24>)  [unwired: 1 in, 1 out]
                        n86 = property class="CameraSettings"(reference=w163, "Exposure"=w161) -> (reference out=w158:refnum<k24>)  [unwired: 1 in, 1 out]
                        n87 = property class="CameraSettings"(reference=w158, "FramesToCapture"=u16 1) -> (reference out=w160:refnum<k24>, error out=w157:errorcluster)  [unwired: 1 in]
                        n88 = property class="CameraSettings"(reference=w160, error in=w157) -> (error out=w153:errorcluster, "XBinning"=→"XBinning":u16, "YBinning"=→"YBinning":u16, "Exposure"=→"Exposure":u32)  [unwired: 1 out]
                        n89 = invoke class="Camera" method="StartSequence"(reference=w165, error in=w153) -> (reference out=w164:refnum<k24>)  [unwired: 1 in, 2 out]
                      }
                    }
                  }
                }
              }
            }
          }
          event "Select Camera": Value Change {
            n90 = event-data() -> ()  [unwired: 1 in, 6 out]
            n91 = local read "Select Camera"() -> (w171:string)
            n92 = local write item#7(w171) -> ()
          }
          event "Open Camera": Value Change {
            n93 = event-data() -> ()  [unwired: 1 in, 6 out]
            n94 = case shown="True" "Open Camera" {
              tunnel: w181 -> [w187 w202]
              tunnel: w180 -> [w186 w200]
              tunnel: [w186 w188] -> w178
              tunnel: [w187 w199] -> w179
              tunnel: [w185 w194] -> w177
              tunnel: w176 -> [w185 w193]
              tunnel: [w184 w192] -> w175
              tunnel: w174 -> [w184 w191]
              tunnel: w173 -> [w183 w189]
              tunnel: [w183 w190] -> w172
              frame False {
              }
              frame True {
                # "check against null string"
                n95 = local read "Camera status"() -> (w198:bool)
                n96 = local read item#7() -> (w201:string)
                n97 = Not Equal?(x=w201, y="") -> (x != y?=w197:bool)
                n98 = Not(x=w198) -> (.not. x?=w196:bool)
                n99 = And(x=w197, y=w196) -> (x .and. y?=w195:bool)
                n100 = case shown="True" w195 {
                  tunnel: w202 -> [w204 w219]
                  tunnel: w201 -> [_ w218]
                  tunnel: [w208 w216] -> w188
                  tunnel: w200 -> [w208 _]
                  tunnel: [w204 w217] -> w199
                  tunnel: [w207 w211] -> w194
                  tunnel: w193 -> [w207 _]
                  tunnel: [w206 w210] -> w192
                  tunnel: w191 -> [w206 _]
                  tunnel: [w205 w209] -> w190
                  tunnel: w189 -> [w205 _]
                  frame False {
                  }
                  frame True {
                    n101 = flat-sequence {
                      tunnel: w219 -> [w228]
                      tunnel: w218 -> [w227]
                      tunnel: [w224] -> w215
                      tunnel: [w223] -> w214
                      tunnel: w215 -> [w292]
                      tunnel: w214 -> [w285]
                      tunnel: [w292] -> w213
                      tunnel: [w247] -> w212
                      tunnel: [w286] -> w211
                      tunnel: [w278] -> w210
                      tunnel: [w272] -> w209
                      tunnel: [w295] -> w216
                      tunnel: [w296] -> w217
                      tunnel: w213 -> [w296]
                      tunnel: w212 -> [w295]
                      frame #0 {
                        n102 = property class="Library"(reference=w228) -> ("Instance"=w221:refnum<k24>)  [unwired: 1 in, 2 out]
                        n103 = invoke class="Library" method="LoadCameras"(reference=w221) -> (reference out=w220:refnum<k24>)  [unwired: 2 in, 2 out]
                        n104 = invoke class="Library" method="GetCamera"(reference=w220, "camName"=w227) -> (reference out=w225:refnum<k24>, "GetCamera"=w226:refnum<k24>)  [unwired: 2 in, 2 out]
                        n105 = Wait (ms)(milliseconds to wait=u32 500) -> ()  [unwired: 1 out]
                        n106 = invoke class="Camera" method="Open"(reference=w226) -> (reference out=w223:refnum<k24>)  [unwired: 2 in, 2 out]
                        n107 = invoke class="Library" method="ShowImage"(reference=w225, "cam"=w223) -> (reference out=w224:refnum<k24>)  [unwired: 2 in, 3 out]
                      }
                      frame #1 {
                        w276 = 0.0 ("upper limit")
                        # "Tiff is1 and Raw is 0"
                        # "Populate settings parameters"
                        # "Register callbacks for\n- Histogram\n- Caputuring indicator\n- Buffer index, Disk queue size, Scroll bar\n- Buffer size"
                        n108 = control-ref of="Post-processing function"() -> (w241:refnum<vi>)
                        n109 = property class="Camera"(reference=w285) -> (reference out=w247:refnum<k24>, "Settings"=w248:refnum<k24>, "AcquisitionBuffer"=w273:refnum<k24>)  [unwired: 1 in, 1 out]
                        n110 = property class="CameraSettings"(reference=w248) -> (reference out=w260:refnum<k24>, error out=w250:errorcluster, "ExposureTime"=w234:refnum<k24>, "SupportedBinning"=w251:refnum<k24>, "ClearCycles"=w261:refnum<k24>, "ClearingModes"=w237:refnum<k24>)  [unwired: 1 in]
                        n111 = control-ref of="Post-processing function value"() -> (w242:refnum<vi>)
                        n112 = control-ref of="Exposure Time"() -> (w230:refnum<vi>)
                        n113 = control-ref of="Capturing"() -> (w284:refnum<vi>)
                        n114 = control-ref of="8 Bit Histogram"() -> (w288:refnum<vi>)
                        n115 = vi-ref "PVCamPropertyChangedCallbackForCameraState.vi"() -> ("vi reference"=w283:refnum<vi>)
                        n116 = vi-ref "PVCamPropertyChangedCallbackForHistogram.vi"() -> ("vi reference"=w287:refnum<vi>)
                        n117 = property class="PmNumericParam`1[[System.UInt64"(reference=w234) -> ("Max"=w233:u64, "Min"=w232:u64, "Current"=w231:u64)  [unwired: 1 in, 2 out]
                        n118 = node(w273, w287, w288) -> (w286:refnum<k27>)  [unwired: 2 in, 1 out]
                        n119 = node(w285, w283, w284) -> (w278:refnum<k27>)  [unwired: 2 in, 1 out]
                        n120 = control-ref of="Disk queue size"() -> (w267:refnum<vi>)
                        n121 = control-ref of="Buffer Index"() -> (w268:refnum<vi>)
                        n122 = vi-ref "PVCamPropertyChangedEventCallbackForBufferIndexQueuedFrames.vi"() -> ("vi reference"=w269:refnum<vi>)
                        n123 = control-ref of="Scrollbar"() -> (w271:refnum<vi>)
                        n124 = In Range and Coerce(upper limit=w233, x=w231, lower limit=w232) -> (coerced(x)=w229:u64)  [unwired: 1 out]
                        n125 = property class="DigNum (strict)"(reference=w230, "Value"=w229) -> ()  [unwired: 1 in, 2 out]
                        n126 = Bundle("Buffer Index"=w268, "Disk queue size"=w267, "Scrollbar"=w271) -> (w270:T1)  [unwired: 1 in]
                        n127 = node ("Register Event Callback")(w273, w269, w270) -> (w272:refnum<k27>)  [unwired: 2 in, 1 out]
                        n128 = control-ref of="Sensor clearing mode"() -> (w236:refnum<vi>)
                        n129 = control-ref of="Binning"() -> (w282:refnum<vi>)
                        n130 = property class="CameraSettings"(reference=w260, error in=w250) -> (reference out=w249:refnum<k24>, "ExposeOutMode"=w259:refnum<k24>, "SpeedTable"=w257:refnum<k24>, "SensorHeight"=w256:refnum<k24>, "SensorWidth"=w255:refnum<k24>)  [unwired: 1 out]
                        n131 = call "PopulateSupportedBinning.vi"("Binning"=w282, ".NET Refnum in"=w251) -> ()  [unwired: 10 in]
                        n132 = call "PopulateClearModes.vi"("ClearingModes"=w237, "ComboBox in"=w236) -> ()  [unwired: 10 in]
                        n133 = property class="AcqBuffer"(reference=w273) -> ("BufferSize"=w266:u32)  [unwired: 1 in, 2 out]
                        n134 = control-ref of="Clear Cycles"() -> (w281:refnum<vi>)
                        n135 = call "PopulateClearCycles.vi"("ClearCycles"=w261, "Digital in"=w281) -> ()  [unwired: 10 in]
                        n136 = control-ref of="Trigger Out Behavior"() -> (w280:refnum<vi>)
                        n137 = In Range and Coerce(upper limit=w266, x=w276, lower limit=w276) -> (coerced(x)=w274:dbl)  [unwired: 1 out]
                        n138 = control-ref of="Scrollbar"() -> (w275:refnum<vi>)
                        n139 = control-ref of="Clearing modes"() -> (w235:refnum<vi>)
                        n140 = control-ref of="Gain"() -> (w291:refnum<vi>)
                        n141 = control-ref of="Readout ports and speeds"() -> (w258:refnum<vi>)
                        n142 = call "SetClearingMode.vi"("Clear mode"=w236, "Clearing modes"=w235, ".NET Refnum in"=w237) -> ()  [unwired: 9 in]
                        n143 = property class="PmNumericParam`1[[System.UInt32"(reference=w255) -> ("Max"=w290:u32)  [unwired: 1 in, 2 out]
                        n144 = property class="PmNumericParam`1[[System.UInt32"(reference=w256) -> ("Max"=w289:u32)  [unwired: 1 in, 2 out]
                        n145 = call "PopulateExpOut.vi"("ExposeOutMode"=w259, "ComboBox in"=w280) -> ()  [unwired: 10 in]
                        n146 = property class="Scroll (strict)"(reference=w275, "Value"=w274, "DocMax"=w266, "DocMin"=0.0 ("Doc Min"), "PageSize"=1.0 ("Page Size")) -> ()  [unwired: 1 in, 2 out]
                        n147 = call "PopulatePortsAndSpeedsGain.vi"("Ports and Speeds"=w258, "Gain"=w291, ".NET Refnum in"=w257) -> ()  [unwired: 9 in]
                        n148 = control-ref of="Bayer pattern"() -> (w263:refnum<vi>)
                        n149 = control-ref of="Name"() -> (w262:refnum<vi>)
                        n150 = control-ref of="Format (0 for RAW[mono only] and 1 for TIFF[mono/color])"() -> (w243:refnum<vi>)
                        n151 = property class="DigNum (strict)"(reference=w243, "Increment"=1.0 ("Data Entry Limits:Increment"), "Maximum"=1.0 ("Data Entry Limits:Maximum"), "Minimum"=0.0 ("Data Entry Limits:Minimum")) -> ()  [unwired: 1 in, 2 out]
                        n152 = property class="CameraSettings"(reference=w249) -> (reference out=w238:refnum<k24>, "ExposureMode"=w254:refnum<k24>, "ExpRes"=w253:refnum<k24>, "ColorMode"=w252:refnum<k24>)  [unwired: 1 in, 1 out]
                        n153 = property class="CameraSettings"(reference=w238) -> (reference out=w240:refnum<k24>, "PpIndex"=w239:refnum<k24>)  [unwired: 1 in, 1 out]
                        n154 = call "PopulatePostProcessing.vi"("Value"=w242, "Post Processing"=w241, "PpIndex"=w239, ".NET Refnum in"=w240) -> ()  [unwired: 8 in]
                        n155 = local write "Full CCD Height"(w289) -> ()
                        n156 = local write "Height"(w289) -> ()
                        n157 = local write "Full CCD Width"(w290) -> ()
                        n158 = local write "Width"(w290) -> ()
                        n159 = call "PopulateColorMode.vi"("Bayer pattern"=w263, "ColorMode"=w252, "String in"=w262) -> ()  [unwired: 9 in]
                        n160 = control-ref of="Trigger In Behavior"() -> (w279:refnum<vi>)
                        n161 = control-ref of="Exposure Resolution"() -> (w277:refnum<vi>)
                        n162 = call "PopulateTriggerModes.vi"("ExposureMode"=w254, "ComboBox in"=w279) -> ()  [unwired: 10 in]
                        n163 = call "PopulateExposureResolution.vi"("Exposure Resolution"=w277, ".NET Refnum in"=w253) -> ()  [unwired: 10 in]
                      }
                      frame #2 {
                        n164 = local write "Camera status"(TRUE ("Camera Status")) -> ()
                        n165 = Wait (ms)(milliseconds to wait=u32 500) -> ()  [unwired: 1 out]
                      }
                    }
                  }
                }
              }
            }
          }
          event "Disk streaming On/Off", "Format (0 for RAW[mono only] and 1 for TIFF[mono/color])": Value Change {
            n166 = event-data() -> ()  [unwired: 1 in, 6 out]
            n167 = local read "Camera status"() -> (w302:bool)
            n168 = case shown="True" w302 {
              tunnel: w301 -> [w303 w307]
              tunnel: [w303 w304] -> w300
              frame False {
              }
              frame True {
                w308 = 0 items=["Idle", "Capturing"] ("Status")
                n169 = property class="Camera"(reference=w307) -> (reference out=w305:refnum<k24>, "IsOpen"=w311:bool, "Status"=w310:i32)  [unwired: 1 in, 1 out]
                n170 = Equal?(x=w311, y=TRUE) -> (x = y?=w312:bool)
                n171 = Equal?(x=w310, y=w308) -> (x = y?=w313:bool)
                n172 = Equal?(x=w312, y=w313) -> (x = y?=w306:bool)
                n173 = case shown="True" w306 {
                  tunnel: w305 -> [w314 w323]
                  tunnel: [w314 w316] -> w304
                  frame False {
                  }
                  frame True {
                    n174 = local read "Format (0 for RAW[mono only] and 1 for TIFF[mono/color])"() -> (w319:u8)
                    n175 = property class="Camera"(reference=w323) -> (reference out=w316:refnum<k24>, "AcquisitionBuffer"=w322:refnum<k24>)  [unwired: 1 in, 1 out]
                    n176 = local read "Disk stream saving path"() -> (w320:string)
                    n177 = local read "Disk streaming On/Off"() -> (w321:bool)
                    n178 = local write "Stream Saving"(w321) -> ()
                    n179 = property class="AcqBuffer"(reference=w322, "DiskStreamingRequired"=w321, "DiskStreamingSavingPath"=w320, "DiskStreamingFormat"=w319) -> (reference out=w318:refnum<k24>)  [unwired: 1 in, 1 out]
                    n180 = property class="AcqBuffer"(reference=w318) -> ("DiskStreamingSavingPath"=w315:string, "DiskStreamingFormat"=w317:u32)  [unwired: 1 in, 2 out]
                    n181 = local write "Format (0 for RAW[mono only] and 1 for TIFF[mono/color])"(w317) -> ()
                    n182 = local write "Disk stream saving path"(w315) -> ()
                    n183 = local write "Image saving path"(w315) -> ()
                  }
                }
              }
            }
          }
          event "Image saving path": Value Change {
            n184 = event-data() -> ()  [unwired: 1 in, 6 out]
            n185 = local read "Camera status"() -> (w329:bool)
            n186 = local read "Image saving path"() -> (w328:path)
            n187 = case shown="True" w329 {
              tunnel: w330 -> [w331 w336]
              tunnel: [w331 w333] -> w324
              tunnel: w328 -> [_ w332]
              frame False {
              }
              frame True {
                w341 = 0 items=["Idle", "Capturing"] ("Status")
                n188 = property class="Camera"(reference=w336) -> (reference out=w334:refnum<k24>, "IsOpen"=w340:bool, "Status"=w342:i32)  [unwired: 1 in, 1 out]
                n189 = Equal?(x=w340, y=TRUE) -> (x = y?=w338:bool)
                n190 = Equal?(x=w342, y=w341) -> (x = y?=w337:bool)
                n191 = Equal?(x=w338, y=w337) -> (x = y?=w335:bool)
                n192 = case shown="True" w335 {
                  tunnel: w334 -> [w344 w350]
                  tunnel: [w344 w349] -> w333
                  tunnel: w332 -> [_ w346]
                  frame False {
                    n193 = One Button Dialog(message="Camera is not idle") -> ()  [unwired: 1 in, 1 out]
                  }
                  frame True {
                    n194 = call <vilib>:"Check if File or Folder Exists.vi"("path"=w346) -> ("file or folder exists?"=w347:bool)  [unwired: 8 in, 2 out]
                    n195 = case shown="True" w347 {
                      tunnel: w346 -> [_ w356]
                      tunnel: ["" w353] -> w345
                      frame False {
                        n196 = One Button Dialog(message="The specified folder doesn't exist") -> ()  [unwired: 1 in, 1 out]
                      }
                      frame True {
                        # "Here we need to append \"\\\" to the path"
                        n197 = Path To String(path=w356) -> (string=w355:string)
                        n198 = Concatenate Strings(w355, "\\" ("string")) -> (w353:string)
                      }
                    }
                    n199 = property class="Camera"(reference=w350) -> (reference out=w349:refnum<k24>, "AcquisitionBuffer"=w348:refnum<k24>)  [unwired: 1 in, 1 out]
                    n200 = property class="AcqBuffer"(reference=w348, "DiskStreamingSavingPath"=w345) -> ()  [unwired: 1 in, 2 out]
                    n201 = local write "Disk stream saving path"(w345) -> ()
                    n202 = local write "Image saving path"(w345) -> ()
                  }
                }
              }
            }
          }
          event "Close Camera": Value Change {
            n203 = event-data() -> ()  [unwired: 1 in, 6 out]
            n204 = case shown="True" "Close Camera" {
              tunnel: w363 -> [w369 w377]
              tunnel: [w369 w378] -> w364
              tunnel: w362 -> [w368 w375]
              tunnel: [w368 w374] -> w361
              tunnel: w360 -> [w367 w373]
              tunnel: [w367 w372] -> w357
              tunnel: w359 -> [w366 w371]
              tunnel: [w366 w370] -> w358
              frame False {
              }
              frame True {
                n205 = local read "Camera status"() -> (w376:bool)
                n206 = case shown="True" w376 {
                  tunnel: [w383 w390] -> w378
                  tunnel: w377 -> [w383 w393]
                  tunnel: w375 -> [w381 w389]
                  tunnel: [w381 w388] -> w374
                  tunnel: w373 -> [w380 w387]
                  tunnel: [w380 w386] -> w372
                  tunnel: w371 -> [w379 w385]
                  tunnel: [w379 w384] -> w370
                  frame False {
                    n207 = One Button Dialog(message="Camera is not open") -> ()  [unwired: 1 in, 1 out]
                  }
                  frame True {
                    w394 = 0 items=["Idle", "Capturing"] ("Status")
                    n208 = property class="Camera"(reference=w393) -> (reference out=w391:refnum<k24>, "IsOpen"=w397:bool, "Status"=w396:i32)  [unwired: 1 in, 1 out]
                    n209 = Equal?(x=w397, y=TRUE) -> (x = y?=w398:bool)
                    n210 = Equal?(x=w396, y=w394) -> (x = y?=w399:bool)
                    n211 = Equal?(x=w398, y=w399) -> (x = y?=w392:bool)
                    n212 = case shown="True" w392 {
                      tunnel: w391 -> [w403 w413]
                      tunnel: [w403 w411] -> w390
                      tunnel: w389 -> [w402 w409]
                      tunnel: [w402 w408] -> w388
                      tunnel: w387 -> [w401 w407]
                      tunnel: [w401 w406] -> w386
                      tunnel: w385 -> [w400 w405]
                      tunnel: [w400 w404] -> w384
                      frame False {
                      }
                      frame True {
                        n213 = flat-sequence {
                          tunnel: w413 -> [w415]
                          tunnel: [w419] -> w412
                          tunnel: w409 -> [w417]
                          tunnel: w407 -> [w416]
                          tunnel: w405 -> [w414]
                          tunnel: w412 -> [w427]
                          tunnel: [w426] -> w410
                          tunnel: [w483] -> w411
                          tunnel: w410 -> [w483]
                          tunnel: [refnum<k27> refnum ("Event Callback")] -> w408
                          tunnel: [refnum<k27> refnum ("Event Callback")] -> w406
                          tunnel: [refnum<k27> refnum ("Event Callback")] -> w404
                          tunnel: [refnum<k27> refnum ("Event Callback")] -> _
                          frame #0 {
                            n214 = Unregister For Events(event registration refnum=w414) -> ()  [unwired: 1 in, 1 out]
                            n215 = property class="Camera"(reference=w415) -> (reference out=w419:refnum<k24>, "Settings"=w423:refnum<k24>)  [unwired: 1 in, 1 out]
                            n216 = Unregister For Events(event registration refnum=w417) -> ()  [unwired: 1 in, 1 out]
                            n217 = Unregister For Events(event registration refnum=w416) -> ()  [unwired: 1 in, 1 out]
                            n218 = property class="CameraSettings"(reference=w423) -> ("Regions"=w422:refnum<k24>)  [unwired: 1 in, 2 out]
                            n219 = property class="PmObservableCollection`1[[PVCam"(reference=w422) -> (reference out=w420:refnum<k24>, "Count"=w421:i32)  [unwired: 1 in, 1 out]
                            n220 = for {
                              N: w421 -> [_]
                              tunnel: w420 -> [w425]
                              i -> [w424]
                              n221 = invoke class="PmObservableCollection`1[[PVCam" method="RemoveAt"(reference=w425, "index"=w424) -> ()  [unwired: 2 in, 4 out]
                            }
                            n222 = Wait (ms)(milliseconds to wait=u32 500) -> ()  [unwired: 1 out]
                          }
                          frame #1 {
                            n223 = invoke class="Camera" method="Close"(reference=w427) -> (reference out=w426:refnum<k24>)  [unwired: 2 in, 2 out]
                          }
                          frame #2 {
                            w449 = 0.0 ("Clear Cycle")
                            w461 = 0 ("Full CCD Y")
                            w462 = u32 1 ("Y Binning")
                            w463 = 0.0 ("Clear Cycle")
                            # "Clear display"
                            n224 = control-ref of="Exposure Resolution"() -> (w452:refnum<vi>)
                            n225 = control-ref of="Sensor clearing mode"() -> (w477:refnum<vi>)
                            n226 = control-ref of="Trigger In Behavior"() -> (w481:refnum<vi>)
                            n227 = control-ref of="Trigger Out Behavior"() -> (w476:refnum<vi>)
                            n228 = local write "X Binning"(w462) -> ()
                            n229 = local write "Y Binning"(w462) -> ()
                            n230 = control-ref of="8 Bit Histogram"() -> (w482:refnum<vi>)
                            n231 = control-ref of="Readout ports and speeds"() -> (w480:refnum<vi>)
                            n232 = property class="CmbBox"(reference=w452, "Strings[]"=string[] [] ("Strings []"), "Value"="") -> ()  [unwired: 1 in, 2 out]
                            n233 = property class="CmbBox"(reference=w477, "Strings[]"=string[] [] ("Strings []"), "Value"="") -> ()  [unwired: 1 in, 2 out]
                            n234 = property class="CmbBox"(reference=w481, "Strings[]"=string[] [] ("Strings []"), "Value"="") -> ()  [unwired: 1 in, 2 out]
                            n235 = property class="CmbBox"(reference=w476, "Strings[]"=string[] [] ("Strings []"), "Value"="") -> ()  [unwired: 1 in, 2 out]
                            n236 = property class="WFGraph (strict)"(reference=w482, "Value"=i32[] []) -> ()  [unwired: 1 in, 2 out]
                            n237 = property class="CmbBox"(reference=w480, "Strings[]"=string[] [] ("Strings []"), "Value"="") -> ()  [unwired: 1 in, 2 out]
                            n238 = control-ref of="Binning"() -> (w478:refnum<vi>)
                            n239 = control-ref of="Gain"() -> (w479:refnum<vi>)
                            n240 = local write "Camera status"(FALSE ("Camera Status")) -> ()
                            n241 = local write "Clear Cycles"(w463) -> ()
                            n242 = local write "Exposure Time"(w463) -> ()
                            n243 = local write "Full CCD Width"(w461) -> ()
                            n244 = local write "X"(w461) -> ()
                            n245 = local write "Full CCD X"(w461) -> ()
                            n246 = local write "Height"(w461) -> ()
                            n247 = local write "Y"(w461) -> ()
                            n248 = local write "Full CCD Height"(w461) -> ()
                            n249 = local write "Width"(w461) -> ()
                            n250 = property class="CmbBox"(reference=w478, "Strings[]"=string[] [] ("Strings []"), "Value"="") -> ()  [unwired: 1 in, 2 out]
                            n251 = property class="CmbBox"(reference=w479, "Strings[]"=string[] [] ("Strings []"), "Value"="") -> ()  [unwired: 1 in, 2 out]
                            n252 = local write "Full CCD Y"(w461) -> ()
                            n253 = local write "Buffer Index"(w449) -> ()
                            n254 = local write "Disk queue size"(w449) -> ()
                            n255 = local write "Live status"(FALSE ("Live")) -> ()
                            n256 = Wait (ms)(milliseconds to wait=u32 500) -> ()  [unwired: 1 out]
                            n257 = control-ref of="Post-processing function"() -> (w446:refnum<vi>)
                            n258 = control-ref of="Post-processing function value"() -> (w448:refnum<vi>)
                            n259 = control-ref of="Bayer pattern"() -> (w439:refnum<vi>)
                            n260 = control-ref of="Color (Off/On)"() -> (w443:refnum<vi>)
                            n261 = property class="DigNum (strict)"(reference=w448, "Value"=0.0) -> ()  [unwired: 1 in, 2 out]
                            n262 = local write "Image saving path"("" ("SavingPath")) -> ()
                            n263 = property class="CmbBox"(reference=w446, "Strings[]"=string[] [] ("Strings []"), "Value"="") -> ()  [unwired: 1 in, 2 out]
                            n264 = property class="Bool (strict)"(reference=w443, "Value"=FALSE) -> ()  [unwired: 1 in, 2 out]
                            n265 = property class="CmbBox"(reference=w439, "Strings[]"=string[] [] ("Strings []"), "Value"="") -> ()  [unwired: 1 in, 2 out]
                            n266 = control-ref of="Stream Saving"() -> (w434:refnum<vi>)
                            n267 = control-ref of="Image saving path"() -> (w436:refnum<vi>)
                            n268 = control-ref of="Disk streaming On/Off"() -> (w432:refnum<vi>)
                            n269 = control-ref of="Disk stream saving path"() -> (w438:refnum<vi>)
                            n270 = control-ref of="Format (0 for RAW[mono only] and 1 for TIFF[mono/color])"() -> (w430:refnum<vi>)
                            n271 = property class="Str"(reference=w438, "Value"="") -> ()  [unwired: 1 in, 2 out]
                            n272 = property class="DigNum (strict)"(reference=w430, "Value"=u8 0) -> ()  [unwired: 1 in, 2 out]
                            n273 = property class="Bool (strict)"(reference=w434, "Value"=FALSE) -> ()  [unwired: 1 in, 2 out]
                            n274 = property class="Bool (strict)"(reference=w432, "Value"=FALSE) -> ()  [unwired: 1 in, 2 out]
                            n275 = property class="Path"(reference=w436, "Value"=path "") -> ()  [unwired: 1 in, 2 out]
                          }
                        }
                      }
                    }
                  }
                }
              }
            }
          }
          event "Get ROI": Value Change {
            n276 = event-data() -> ()  [unwired: 1 in, 6 out]
            n277 = case shown="True" "Get ROI" {
              tunnel: w488 -> [w490 w493]
              tunnel: [w490 w492] -> w484
              frame False {
              }
              frame True {
                n278 = local read "Camera status"() -> (w491:bool)
                n279 = case shown="True" w491 {
                  tunnel: w493 -> [w494 w498]
                  tunnel: [w494 w496] -> w492
                  frame False {
                    n280 = One Button Dialog(message="Camera is not open") -> ()  [unwired: 1 in, 1 out]
                  }
                  frame True {
                    w504 = 0 items=["Idle", "Capturing"] ("Status")
                    n281 = property class="Camera"(reference=w498) -> (reference out=w497:refnum<k24>, "IsOpen"=w503:bool, "Status"=w505:i32)  [unwired: 1 in, 1 out]
                    n282 = Equal?(x=w503, y=TRUE) -> (x = y?=w501:bool)
                    n283 = Equal?(x=w505, y=w504) -> (x = y?=w500:bool)
                    n284 = Equal?(x=w501, y=w500) -> (x = y?=w499:bool)
                    n285 = case shown="True" w499 {
                      tunnel: [w506 w512] -> w496
                      tunnel: w497 -> [w506 w514]
                      frame False {
                      }
                      frame True {
                        n286 = property class="Camera"(reference=w514) -> (reference out=w512:refnum<k24>, "Settings"=w513:refnum<k24>)  [unwired: 1 in, 1 out]
                        n287 = property class="CameraSettings"(reference=w513) -> ("Regions"=w511:refnum<k24>)  [unwired: 1 in, 2 out]
                        n288 = property class="PmObservableCollection`1[[PVCam"(reference=w511) -> (reference out=w507:refnum<k24>, "Count"=w510:i32)  [unwired: 1 in, 1 out]
                        n289 = Greater?(x=w510, y=0) -> (0:w508:bool)
                        n290 = case shown="True" w508 {
                          tunnel: w507 -> [_ w516]
                          frame False {
                            n291 = One Button Dialog(message="ROI isn't created yet") -> ()  [unwired: 1 in, 1 out]
                          }
                          frame True {
                            n292 = invoke class="PmObservableCollection`1[[PVCam" method="get_Item"(reference=w516, "index"=0) -> ("get_Item"=w521:refnum<k24>)  [unwired: 2 in, 3 out]
                            n293 = property class="PmRegion"(reference=w521) -> ("Height"=w520:u16, "Y"=w519:u16, "Width"=w518:u16, "X"=w517:u16)  [unwired: 1 in, 2 out]
                            n294 = local write "Height"(w520) -> ()
                            n295 = local write "Y"(w519) -> ()
                            n296 = local write "Width"(w518) -> ()
                            n297 = local write "X"(w517) -> ()
                          }
                        }
                      }
                    }
                  }
                }
              }
            }
          }
          event "Exposure Time", "Binning", "Sensor clearing mode", "Clear Cycles", "Trigger In Behavior", "Exposure Resolution", "Post-processing function", "Color (Off/On)", "Trigger Out Behavior": Value Change {
            n298 = event-data() -> ()  [unwired: 1 in, 6 out]
            n299 = local read "Camera status"() -> (w527:bool)
            n300 = case shown="True" w527 {
              tunnel: [w530 w532] -> w528
              tunnel: w526 -> [w530 w531]
              frame False {
                n301 = One Button Dialog(message="Camera is not open") -> ()  [unwired: 1 in, 1 out]
              }
              frame True {
                w539 = 0 items=["Idle", "Capturing"] ("Status")
                n302 = property class="Camera"(reference=w531) -> (reference out=w533:refnum<k24>, "IsOpen"=w538:bool, "Status"=w540:i32)  [unwired: 1 in, 1 out]
                n303 = Equal?(x=w538, y=TRUE) -> (x = y?=w536:bool)
                n304 = Equal?(x=w540, y=w539) -> (x = y?=w535:bool)
                n305 = Equal?(x=w536, y=w535) -> (x = y?=w534:bool)
                n306 = case shown="True" w534 {
                  tunnel: w533 -> [w541 w584]
                  tunnel: [w541 w583] -> w532
                  frame False {
                  }
                  frame True {
                    # "Exposure time setting"
                    n307 = property class="Camera"(reference=w584) -> (reference out=w583:refnum<k24>, "Settings"=w582:refnum<k24>)  [unwired: 1 in, 1 out]
                    n308 = property class="CameraSettings"(reference=w582) -> (reference out=w547:refnum<k24>, "ExposureTime"=w552:refnum<k24>, "SupportedBinning"=w579:refnum<k24>, "ClearingModes"=w581:refnum<k24>, "ClearCycles"=w580:refnum<k24>)  [unwired: 1 in, 1 out]
                    n309 = control-ref of="Clearing modes"() -> (w575:refnum<vi>)
                    n310 = control-ref of="Sensor clearing mode"() -> (w573:refnum<vi>)
                    n311 = control-ref of="Clear Cycles"() -> (w570:refnum<vi>)
                    n312 = control-ref of="CC Max"() -> (w568:refnum<vi>)
                    n313 = control-ref of="CC Min"() -> (w569:refnum<vi>)
                    n314 = call "SetClearCycles.vi"("CC Max"=w568, "CC Min"=w569, "Clear Cycle"=w570, ".NET Refnum in"=w580) -> ()  [unwired: 8 in]
                    n315 = call "SetClearingMode.vi"("Clear mode"=w573, "Clearing modes"=w575, ".NET Refnum in"=w581) -> ()  [unwired: 9 in]
                    n316 = control-ref of="Exposure Time"() -> (w549:refnum<vi>)
                    n317 = property class="PmNumericParam`1[[System.UInt64"(reference=w552) -> (reference out=w546:refnum<k24>, "Max"=w551:u64, "Min"=w550:u64)  [unwired: 1 in, 1 out]
                    n318 = property class="DigNum (strict)"(reference=w549) -> (reference out=w543:refnum<vi>, "Value"=w548:dbl)  [unwired: 1 in, 1 out]
                    n319 = control-ref of="Y Binning"() -> (w576:refnum<vi>)
                    n320 = control-ref of="X Binning"() -> (w577:refnum<vi>)
                    n321 = control-ref of="Binning"() -> (w578:refnum<vi>)
                    n322 = call "SetBinning.vi"("SupportedBinning"=w579, "Y Binning"=w576, "Settings"=w547, "X Binning"=w577, "ComboBox in"=w578) -> ()  [unwired: 7 in]
                    n323 = In Range and Coerce(upper limit=w551, x=w548, lower limit=w550) -> (coerced(x)=w544:dbl)  [unwired: 1 out]
                    n324 = control-ref of="Post-processing function"() -> (w553:refnum<vi>)
                    n325 = control-ref of="Post-processing function value"() -> (w554:refnum<vi>)
                    n326 = property class="CameraSettings"(reference=w547, "Exposure"=w544) -> ()  [unwired: 1 in, 2 out]
                    n327 = property class="PmNumericParam`1[[System.UInt64"(reference=w546, "Current"=w544) -> (reference out=w545:refnum<k24>)  [unwired: 1 in, 1 out]
                    n328 = property class="PmNumericParam`1[[System.UInt64"(reference=w545) -> ("Current"=w542:u64)  [unwired: 1 in, 2 out]
                    n329 = control-ref of="Trigger Out Behavior"() -> (w572:refnum<vi>)
                    n330 = control-ref of="Exp. out"() -> (w566:refnum<vi>)
                    n331 = property class="CameraSettings"(reference=w547) -> (reference out=w557:refnum<k24>, "ExposeOutMode"=w561:refnum<k24>, "ExposureMode"=w560:refnum<k24>, "ExpRes"=w559:refnum<k24>)  [unwired: 1 in, 1 out]
                    n332 = property class="CameraSettings"(reference=w557) -> (reference out=w555:refnum<k24>, "PpIndex"=w556:refnum<k24>, "ColorMode"=w558:refnum<k24>)  [unwired: 1 in, 1 out]
                    n333 = call "SetExpOut.vi"("Exp. in"=w572, "ExposeOutMode"=w561, "Digital in"=w566) -> ()  [unwired: 9 in]
                    n334 = control-ref of="Exposure Resolution"() -> (w567:refnum<vi>)
                    n335 = control-ref of="Exposure Resolution"() -> (w565:refnum<vi>)
                    n336 = control-ref of="Color (Off/On)"() -> (w562:refnum<vi>)
                    n337 = control-ref of="Bayer pattern"() -> (w564:refnum<vi>)
                    n338 = control-ref of="Trigger In Behavior"() -> (w571:refnum<vi>)
                    n339 = control-ref of="Trigger Mode"() -> (w574:refnum<vi>)
                    n340 = control-ref of="Name"() -> (w563:refnum<vi>)
                    n341 = property class="DigNum (strict)"(reference=w543, "Value"=w542) -> ()  [unwired: 1 in, 2 out]
                    n342 = call "SetColorMode.vi"("Name"=w563, "Bayer pattern"=w564, "Color (Off/On)"=w562, ".NET Refnum in"=w558) -> ()  [unwired: 8 in]
                    n343 = call "SetExposureResolution.vi"("ExpRes"=w559, "Exposure Resolution"=w567, "ComboBox in"=w565) -> ()  [unwired: 9 in]
                    n344 = call "SetTriggerMode.vi"("Trigger"=w571, "ExposureMode"=w560, "Digital in"=w574) -> ()  [unwired: 9 in]
                    n345 = call "SetPostProcessing.vi"("Post Processing"=w553, "Value"=w554, "PpIndex"=w556, ".NET Refnum in"=w555) -> ()  [unwired: 8 in]
                  }
                }
              }
            }
          }
          event "Readout ports and speeds": Value Change {
            n346 = event-data() -> ()  [unwired: 1 in, 6 out]
            n347 = local read "Camera status"() -> (w590:bool)
            n348 = case shown="True" w590 {
              tunnel: w589 -> [w592 w602]
              tunnel: [w592 w593] -> w585
              frame False {
                n349 = One Button Dialog(message="Camera is not open") -> ()  [unwired: 1 in, 1 out]
              }
              frame True {
                w594 = 0 items=["Idle", "Capturing"] ("Status")
                n350 = property class="Camera"(reference=w602) -> (reference out=w601:refnum<k24>, "IsOpen"=w600:bool, "Status"=w598:i32)  [unwired: 1 in, 1 out]
                n351 = Equal?(x=TRUE, y=w600) -> (x = y?=w596:bool)
                n352 = Equal?(x=w598, y=w594) -> (x = y?=w597:bool)
                n353 = Equal?(x=w596, y=w597) -> (x = y?=w595:bool)
                n354 = case shown="True" w595 {
                  tunnel: w601 -> [w603 w609]
                  tunnel: [w603 w604] -> w593
                  frame False {
                  }
                  frame True {
                    n355 = property class="Camera"(reference=w609) -> (reference out=w604:refnum<k24>, "Settings"=w608:refnum<k24>)  [unwired: 1 in, 1 out]
                    n356 = property class="CameraSettings"(reference=w608) -> ("SpeedTable"=w607:refnum<k24>)  [unwired: 1 in, 2 out]
                    n357 = control-ref of="Readout ports and speeds"() -> (w605:refnum<vi>)
                    n358 = control-ref of="Gain"() -> (w606:refnum<vi>)
                    n359 = call "SetPortsAndSpeedsGain.vi"("Ports and Speeds"=w605, "SpeedTable"=w607, "ComboBox in"=w606) -> ()  [unwired: 9 in]
                  }
                }
              }
            }
          }
          event "Save Image to TIFF": Value Change {
            n360 = event-data() -> ()  [unwired: 1 in, 6 out]
            n361 = case shown="True" "Save Image to TIFF" {
              tunnel: w614 -> [w616 w618]
              tunnel: [w616 w617] -> w613
              frame False {
              }
              frame True {
                n362 = local read "Camera status"() -> (w619:bool)
                n363 = case shown="True" w619 {
                  tunnel: w618 -> [w620 w624]
                  tunnel: [w620 w621] -> w617
                  frame False {
                  }
                  frame True {
                    w625 = 0 items=["Idle", "Capturing"] ("Status")
                    n364 = property class="Camera"(reference=w624) -> (reference out=w622:refnum<k24>, "IsOpen"=w628:bool, "Status"=w627:i32)  [unwired: 1 in, 1 out]
                    n365 = Equal?(x=w628, y=TRUE) -> (x = y?=w629:bool)
                    n366 = Equal?(x=w627, y=w625) -> (x = y?=w630:bool)
                    n367 = Equal?(x=w629, y=w630) -> (x = y?=w623:bool)
                    n368 = case shown="True" w623 {
                      tunnel: w622 -> [w632 w639]
                      tunnel: [w632 w638] -> w621
                      frame False {
                        n369 = One Button Dialog(message="Camera must be idle") -> ()  [unwired: 1 in, 1 out]
                      }
                      frame True {
                        n370 = local read "Disk stream saving path"() -> (w633:string)
                        n371 = String Length(string=w633) -> (length=w636:i32)
                        n372 = Greater?(x=w636, y=0) -> (0:w635:bool)
                        n373 = property class="Camera"(reference=w639) -> (reference out=w638:refnum<k24>, "AcquisitionBuffer"=w634:refnum<k24>)  [unwired: 1 in, 1 out]
                        n374 = case shown="True" w635 {
                          tunnel: w634 -> [_ w643]
                          tunnel: w633 -> [_ w642]
                          frame False {
                            (unwired) "OK"
                            n375 = One Button Dialog(message="Define path for image saving first", button name ("OK")="OK") -> ()  [unwired: 1 out]
                          }
                          frame True {
                            n376 = property class="AcqBuffer"(reference=w643, "ImageSavingPath"=w642) -> (reference out=w646:refnum<k24>)  [unwired: 1 in, 1 out]
                            n377 = property class="AcqBuffer"(reference=w646) -> (reference out=w645:refnum<k24>, "BufferIndex"=w644:u32)  [unwired: 1 in, 1 out]
                            n378 = invoke class="AcqBuffer" method="SaveAsTiff"(reference=w645, "nth"=w644) -> ()  [unwired: 2 in, 4 out]
                          }
                        }
                      }
                    }
                  }
                }
              }
            }
          }
          event "Scrollbar": Value Change {
            n379 = event-data() -> ()  [unwired: 1 in, 6 out]
            n380 = local read "Scrollbar"() -> (w647:i32)
            n381 = local read "Camera status"() -> (w648:bool)
            n382 = case shown="True" w648 {
              tunnel: w653 -> [w654 w660]
              tunnel: [w654 w658] -> w652
              tunnel: w647 -> [_ w656]
              frame False {
                n383 = One Button Dialog(message="Camera is not open") -> ()  [unwired: 1 in, 1 out]
              }
              frame True {
                w665 = 0 items=["Idle", "Capturing"] ("Status")
                n384 = property class="Camera"(reference=w660) -> (reference out=w659:refnum<k24>, "IsOpen"=w664:bool, "Status"=w666:i32)  [unwired: 1 in, 1 out]
                n385 = Equal?(x=w664, y=TRUE) -> (x = y?=w662:bool)
                n386 = Equal?(x=w666, y=w665) -> (x = y?=w661:bool)
                n387 = Equal?(x=w662, y=w661) -> (x = y?=w657:bool)
                n388 = case shown="True" w657 {
                  tunnel: w659 -> [w667 w675]
                  tunnel: [w667 w674] -> w658
                  tunnel: w656 -> [_ w668]
                  frame False {
                  }
                  frame True {
                    n389 = property class="Camera"(reference=w675) -> (reference out=w674:refnum<k24>, "AcquisitionBuffer"=w671:refnum<k24>)  [unwired: 1 in, 1 out]
                    n390 = property class="AcqBuffer"(reference=w671) -> (reference out=w670:refnum<k24>, "BufferSize"=w673:u32)  [unwired: 1 in, 1 out]
                    n391 = In Range and Coerce(upper limit=w673, x=w668, lower limit=0) -> (coerced(x)=w669:u32)  [unwired: 1 out]
                    n392 = property class="AcqBuffer"(reference=w670, "BufferIndex"=w669) -> ()  [unwired: 1 in, 2 out]
                  }
                }
              }
            }
          }
          event "Gain": Value Change {
            n393 = event-data() -> ()  [unwired: 1 in, 6 out]
            n394 = local read "Camera status"() -> (w681:bool)
            n395 = case shown="False" w681 {
              tunnel: w680 -> [w683 w686]
              tunnel: [w683 w684] -> w679
              frame False {
                n396 = One Button Dialog(message="Camera is not open") -> ()  [unwired: 1 in, 1 out]
              }
              frame True {
                w688 = 0 items=["Idle", "Capturing"] ("Status")
                n397 = property class="Camera"(reference=w686) -> (reference out=w685:refnum<k24>, "IsOpen"=w691:bool, "Status"=w690:i32)  [unwired: 1 in, 1 out]
                n398 = Equal?(x=w691, y=TRUE) -> (x = y?=w692:bool)
                n399 = Equal?(x=w690, y=w688) -> (x = y?=w693:bool)
                n400 = Equal?(x=w692, y=w693) -> (x = y?=w687:bool)
                n401 = case shown="True" w687 {
                  tunnel: w685 -> [w694 w697]
                  tunnel: [w694 w696] -> w684
                  frame False {
                  }
                  frame True {
                    n402 = control-ref of="Gain"() -> (w695:refnum<vi>)
                    n403 = call "SetGain.vi"("Gain"=w695, ".NET Refnum in"=w697) -> (".NET Refnum out"=w696:refnum<k24>)  [unwired: 9 in]
                  }
                }
              }
            }
          }
          event "Post-processing function value": Value Change {
            n404 = event-data() -> ()  [unwired: 1 in, 6 out]
            n405 = local read "Camera status"() -> (w703:bool)
            n406 = case shown="True" w703 {
              tunnel: w702 -> [w705 w709]
              tunnel: [w705 w706] -> w701
              frame False {
                n407 = One Button Dialog(message="Camera is not open") -> ()  [unwired: 1 in, 1 out]
              }
              frame True {
                w710 = 0 items=["Idle", "Capturing"] ("Status")
                n408 = property class="Camera"(reference=w709) -> (reference out=w707:refnum<k24>, "IsOpen"=w713:bool, "Status"=w712:i32)  [unwired: 1 in, 1 out]
                n409 = Equal?(x=w713, y=TRUE) -> (x = y?=w714:bool)
                n410 = Equal?(x=w712, y=w710) -> (x = y?=w715:bool)
                n411 = Equal?(x=w714, y=w715) -> (x = y?=w708:bool)
                n412 = case shown="True" w708 {
                  tunnel: w707 -> [w716 w722]
                  tunnel: [w716 w717] -> w706
                  frame False {
                  }
                  frame True {
                    n413 = property class="Camera"(reference=w722) -> (reference out=w717:refnum<k24>, "Settings"=w721:refnum<k24>)  [unwired: 1 in, 1 out]
                    n414 = property class="CameraSettings"(reference=w721) -> ("PpIndex"=w720:refnum<k24>, "PpParam"=w718:refnum<k24>)  [unwired: 1 in, 2 out]
                    n415 = property class="PmNumericSpecialParam`1[[System"(reference=w720) -> ("Available"=w719:bool)  [unwired: 1 in, 2 out]
                    n416 = case shown="True" w719 {
                      tunnel: w718 -> [_ w728]
                      frame False {
                      }
                      frame True {
                        # "1. Check if the input is in the right range\n2. Set the input value\n3. Display the set value"
                        n417 = control-ref of="Post-processing function value"() -> (w732:refnum<vi>)
                        n418 = property class="PmPostProcessingParam"(reference=w728) -> (reference out=w726:refnum<k24>, "Max"=w730:u32, "Min"=w729:u32)  [unwired: 1 in, 1 out]
                        n419 = property class="DigNum (strict)"(reference=w732) -> (reference out=w725:refnum<vi>, "Value"=w731:dbl)  [unwired: 1 in, 1 out]
                        n420 = In Range and Coerce(upper limit=w730, x=w731, lower limit=w729) -> (coerced(x)=w727:dbl)  [unwired: 1 out]
                        n421 = property class="PmPostProcessingParam"(reference=w726, "Current"=w727) -> (reference out=w723:refnum<k24>)  [unwired: 1 in, 1 out]
                        n422 = property class="PmPostProcessingParam"(reference=w723) -> ("Current"=w724:u32)  [unwired: 1 in, 2 out]
                        n423 = property class="DigNum (strict)"(reference=w725, "Value"=w724) -> ()  [unwired: 1 in, 2 out]
                      }
                    }
                  }
                }
              }
            }
          }
          event "Y", "X", "Width", "Height": Value Change {
            n424 = event-data() -> ()  [unwired: 1 in, 6 out]
            n425 = local read "Camera status"() -> (w737:bool)
            n426 = case shown="True" w737 {
              tunnel: w738 -> [w739 w744]
              tunnel: [w739 w741] -> w734
              frame False {
                n427 = One Button Dialog(message="Camera is not open") -> ()  [unwired: 1 in, 1 out]
              }
              frame True {
                w749 = 0 items=["Idle", "Capturing"] ("Status")
                n428 = property class="Camera"(reference=w744) -> (reference out=w742:refnum<k24>, "IsOpen"=w748:bool, "Status"=w750:i32)  [unwired: 1 in, 1 out]
                n429 = Equal?(x=w748, y=TRUE) -> (x = y?=w746:bool)
                n430 = Equal?(x=w750, y=w749) -> (x = y?=w745:bool)
                n431 = Equal?(x=w746, y=w745) -> (x = y?=w743:bool)
                n432 = case shown="True" w743 {
                  tunnel: w742 -> [w751 w754]
                  tunnel: [w751 w753] -> w741
                  frame False {
                  }
                  frame True {
                    n433 = flat-sequence {
                      tunnel: w754 -> [w755]
                      tunnel: [w755] -> w752
                      tunnel: [w797] -> w753
                      tunnel: w752 -> [w804]
                      frame #0 {
                        # "if (!( x >= 0\n            && (x+width) <= full_width\n            &&  0 < width \n            && y >= 0\n            && (y+height) <= full_height\n            && 0 < height ))\n        {\n           printf(\"Incorrect range for a ROI. \\n\");\n        }"
                        # "1. Check ROI \n2. Set ROI"
                        n434 = local read "Width"() -> (w783:u16)
                        n435 = local read "Full CCD Width"() -> (w767:i32)
                        n436 = local read "X"() -> (w784:u16)
                        n437 = local read "Width"() -> (w764:u16)
                        n438 = Add(x=w784, y=w783) -> (x+y=w766:u16)
                        n439 = local read "Height"() -> (w780:u16)
                        n440 = Less Or Equal?(x=w766, y=w767) -> (x <= y?=w777:bool)
                        n441 = local read "Full CCD Height"() -> (w763:i32)
                        n442 = Less?(x=u16 0, y=w764) -> (x < y?=w776:bool)
                        n443 = local read "X"() -> (w786:u16)
                        n444 = local read "Y"() -> (w781:u16)
                        n445 = local read "Y"() -> (w779:u16)
                        n446 = local read "Height"() -> (w760:u16)
                        n447 = Greater Or Equal?(x=w786, y=u16 0) -> (x >= y?=w778:bool)
                        n448 = Greater Or Equal?(x=w781, y=u16 0) -> (x >= y?=w775:bool)
                        n449 = Add(x=w780, y=w779) -> (x+y=w762:u16)
                        n450 = Less Or Equal?(x=w762, y=w763) -> (x <= y?=w774:bool)
                        n451 = And(x=w778, y=w777) -> (x .and. y?=w772:bool)
                        n452 = And(x=w776, y=w775) -> (x .and. y?=w771:bool)
                        n453 = Less?(x=u16 0, y=w760) -> (x < y?=w773:bool)
                        n454 = And(x=w772, y=w771) -> (x .and. y?=w770:bool)
                        n455 = And(x=w774, y=w773) -> (x .and. y?=w769:bool)
                        n456 = And(x=w770, y=w769) -> (x .and. y?=w768:bool)
                        n457 = case shown="False" w768 {
                          tunnel: [w788 w795] -> w759
                          tunnel: [u16 0 ("X") w794] -> w757
                          tunnel: [u16 0 ("Y") w793] -> w758
                          tunnel: [w789 w792] -> w756
                          frame False {
                            n458 = local read "Full CCD Height"() -> (w789:i32)
                            n459 = local read "Full CCD Width"() -> (w788:i32)
                            n460 = One Button Dialog(message="Wrong ROI ! Resetting to full CCD") -> ()  [unwired: 1 in, 1 out]
                          }
                          frame True {
                            n461 = local read "Height"() -> (w792:u16)
                            n462 = local read "Width"() -> (w795:u16)
                            n463 = local read "Y"() -> (w793:u16)
                            n464 = local read "X"() -> (w794:u16)
                          }
                        }
                        n465 = local write "Y"(w758) -> ()
                        n466 = local write "X"(w757) -> ()
                        n467 = local write "Width"(w759) -> ()
                        n468 = local write "Height"(w756) -> ()
                      }
                      frame #1 {
                        n469 = property class="Camera"(reference=w804) -> (reference out=w797:refnum<k24>, error out=w803:errorcluster, "Settings"=w802:refnum<k24>)  [unwired: 1 in]
                        n470 = property class="CameraSettings"(reference=w802, error in=w803) -> ("Regions"=w801:refnum<k24>)  [unwired: 2 out]
                        n471 = property class="PmObservableCollection`1[[PVCam"(reference=w801) -> (reference out=w796:refnum<k24>, "Count"=w799:i32)  [unwired: 1 in, 1 out]
                        n472 = Greater?(x=w799, y=0) -> (0:w798:bool)
                        n473 = case shown="True" w798 {
                          tunnel: w796 -> [_ w806]
                          frame False {
                            n474 = One Button Dialog(message="ROI is not created.") -> ()  [unwired: 1 in, 1 out]
                          }
                          frame True {
                            # "Display ROI"
                            n475 = invoke class="PmObservableCollection`1[[PVCam" method="get_Item"(reference=w806, "index"=0) -> ("get_Item"=w808:refnum<k24>)  [unwired: 2 in, 3 out]
                            n476 = local read "Height"() -> (w809:u16)
                            n477 = local read "Width"() -> (w810:u16)
                            n478 = local read "X"() -> (w811:u16)
                            n479 = local read "Y"() -> (w812:u16)
                            n480 = property class="PmRegion"(reference=w808, "Height"=w809, "Width"=w810, "X"=w811, "Y"=w812) -> ()  [unwired: 1 in, 2 out]
                          }
                        }
                      }
                    }
                  }
                }
              }
            }
          }
          event "Full CCD": Value Change {
            n481 = event-data() -> ()  [unwired: 1 in, 6 out]
            n482 = case shown="True" "Full CCD" {
              tunnel: w818 -> [w819 w822]
              tunnel: [w819 w821] -> w817
              frame False {
              }
              frame True {
                n483 = local read "Camera status"() -> (w820:bool)
                n484 = case shown="True" w820 {
                  tunnel: w822 -> [w824 w828]
                  tunnel: [w824 w826] -> w821
                  frame False {
                    n485 = One Button Dialog(message="Camera is not open") -> ()  [unwired: 1 in, 1 out]
                  }
                  frame True {
                    w833 = 0 items=["Idle", "Capturing"] ("Status")
                    n486 = property class="Camera"(reference=w828) -> (reference out=w825:refnum<k24>, "IsOpen"=w832:bool, "Status"=w834:i32)  [unwired: 1 in, 1 out]
                    n487 = Equal?(x=w832, y=TRUE) -> (x = y?=w830:bool)
                    n488 = Equal?(x=w834, y=w833) -> (x = y?=w829:bool)
                    n489 = Equal?(x=w830, y=w829) -> (x = y?=w827:bool)
                    n490 = case shown="True" w827 {
                      tunnel: [w835 w843] -> w826
                      tunnel: w825 -> [w835 w844]
                      frame False {
                      }
                      frame True {
                        n491 = property class="Camera"(reference=w844) -> (reference out=w843:refnum<k24>, "Settings"=w842:refnum<k24>)  [unwired: 1 in, 1 out]
                        n492 = property class="CameraSettings"(reference=w842) -> (reference out=w836:refnum<k24>, "Regions"=w841:refnum<k24>)  [unwired: 1 in, 1 out]
                        n493 = property class="PmObservableCollection`1[[PVCam"(reference=w841) -> (reference out=w837:refnum<k24>, "Count"=w840:i32)  [unwired: 1 in, 1 out]
                        n494 = Greater?(x=w840, y=0) -> (0:w838:bool)
                        n495 = case shown="True" w838 {
                          tunnel: w837 -> [_ w853]
                          tunnel: w836 -> [_ w852]
                          frame False {
                            n496 = One Button Dialog(message="ROI is not created.") -> ()  [unwired: 1 in, 1 out]
                          }
                          frame True {
                            n497 = invoke class="PmObservableCollection`1[[PVCam" method="RemoveAt"(reference=w853, "index"=0) -> ()  [unwired: 2 in, 4 out]
                            n498 = property class="CameraSettings"(reference=w852) -> ("SensorWidth"=w851:refnum<k24>)  [unwired: 1 in, 2 out]
                            n499 = property class="CameraSettings"(reference=w852) -> ("SensorHeight"=w850:refnum<k24>)  [unwired: 1 in, 2 out]
                            n500 = property class="PmNumericParam`1[[System.UInt32"(reference=w851) -> ("Current"=w849:u32)  [unwired: 1 in, 2 out]
                            n501 = property class="PmNumericParam`1[[System.UInt32"(reference=w850) -> ("Current"=w848:u32)  [unwired: 1 in, 2 out]
                            n502 = local write "Width"(w849) -> ()
                            n503 = local write "Height"(w848) -> ()
                            n504 = local write "X"(0 ("index")) -> ()
                            n505 = local write "Y"(0 ("index")) -> ()
                          }
                        }
                      }
                    }
                  }
                }
              }
            }
          }
          event "Live start": Value Change {
            n506 = event-data() -> ()  [unwired: 1 in, 6 out]
            n507 = case shown="True" "Live start" {
              tunnel: w859 -> [w861 w864]
              tunnel: [w861 w863] -> w858
              frame False {
              }
              frame True {
                n508 = local read "Camera status"() -> (w862:bool)
                n509 = case shown="True" w862 {
                  tunnel: w864 -> [w866 w870]
                  tunnel: [w866 w867] -> w863
                  frame False {
                    n510 = One Button Dialog(message="Camera is not open") -> ()  [unwired: 1 in, 1 out]
                  }
                  frame True {
                    w875 = 0 items=["Idle", "Capturing"] ("Status")
                    n511 = property class="Camera"(reference=w870) -> (reference out=w868:refnum<k24>, "IsOpen"=w874:bool, "Status"=w876:i32)  [unwired: 1 in, 1 out]
                    n512 = Equal?(x=w874, y=TRUE) -> (x = y?=w872:bool)
                    n513 = Equal?(x=w876, y=w875) -> (x = y?=w871:bool)
                    n514 = Equal?(x=w872, y=w871) -> (x = y?=w869:bool)
                    n515 = case shown="True" w869 {
                      tunnel: w868 -> [w877 w883]
                      tunnel: [w877 w885] -> w867
                      frame False {
                      }
                      frame True {
                        n516 = control-ref of="Exposure Time"() -> (w879:refnum<vi>)
                        n517 = local write "Live status"(TRUE ("Live")) -> ()
                        n518 = property class="DigNum (strict)"(reference=w879) -> ("Value"=w878:dbl)  [unwired: 1 in, 2 out]
                        n519 = property class="Camera"(reference=w883) -> (reference out=w882:refnum<k24>, "Settings"=w881:refnum<k24>)  [unwired: 1 in, 1 out]
                        n520 = property class="CameraSettings"(reference=w881, "Exposure"=w878) -> (error out=w880:errorcluster)  [unwired: 1 in, 1 out]
                        n521 = invoke class="Camera" method="StartLive"(reference=w882, error in=w880) -> (reference out=w885:refnum<k24>)  [unwired: 1 in, 2 out]
                      }
                    }
                  }
                }
              }
            }
          }
          event "Live stop": Value Change {
            n522 = event-data() -> ()  [unwired: 1 in, 6 out]
            n523 = case shown="True" "Live stop" {
              tunnel: w890 -> [w892 w895]
              tunnel: [w892 w894] -> w889
              frame False {
              }
              frame True {
                n524 = local read "Camera status"() -> (w893:bool)
                n525 = case shown="True" w893 {
                  tunnel: w895 -> [w896 w901]
                  tunnel: [w896 w899] -> w894
                  frame False {
                    n526 = One Button Dialog(message="Camera is not open") -> ()  [unwired: 1 in, 1 out]
                  }
                  frame True {
                    w906 = 1 items=["Idle", "Capturing"] ("Status")
                    n527 = property class="Camera"(reference=w901) -> (reference out=w900:refnum<k24>, "IsOpen"=w905:bool, "Status"=w907:i32)  [unwired: 1 in, 1 out]
                    n528 = Equal?(x=w907, y=w906) -> (x = y?=w902:bool)
                    n529 = Equal?(x=w905, y=TRUE) -> (x = y?=w903:bool)
                    n530 = Equal?(x=w903, y=w902) -> (x = y?=w898:bool)
                    n531 = case shown="True" w898 {
                      tunnel: w900 -> [w908 w911]
                      tunnel: [w908 w910] -> w899
                      frame False {
                      }
                      frame True {
                        n532 = invoke class="Camera" method="Stop"(reference=w911) -> (reference out=w910:refnum<k24>)  [unwired: 2 in, 2 out]
                        n533 = local write "Live status"(FALSE ("Live")) -> ()
                      }
                    }
                  }
                }
              }
            }
          }
          event "Histogram On/Off": Value Change {
            n534 = event-data() -> ()  [unwired: 1 in, 6 out]
            n535 = local read "Camera status"() -> (w912:bool)
            n536 = case shown="True" w912 {
              tunnel: w915 -> [w920 w922]
              tunnel: [w920 w925] -> w914
              tunnel: "Histogram On/Off" -> [_ w924]
              frame False {
                n537 = One Button Dialog(message="Camera is not open") -> ()  [unwired: 1 in, 1 out]
              }
              frame True {
                n538 = property class="Camera"(reference=w922) -> (reference out=w923:refnum<k24>, "IsOpen"=w921:bool)  [unwired: 1 in, 1 out]
                n539 = case shown="True" w921 {
                  tunnel: w923 -> [w926 w929]
                  tunnel: [w926 w928] -> w925
                  tunnel: w924 -> [_ w927]
                  frame False {
                  }
                  frame True {
                    n540 = global write "PVCamGlobalVariables.vi" "Histogram Enabled"(w927) -> ()
                    n541 = property class="Camera"(reference=w929) -> (reference out=w928:refnum<k24>, "AcquisitionBuffer"=w930:refnum<k24>)  [unwired: 1 in, 1 out]
                    n542 = property class="AcqBuffer"(reference=w930, "UseScaling"=w927) -> ()  [unwired: 1 in, 2 out]
                  }
                }
              }
            }
          }
        }
      }
    }
    frame #2 {
      # "Library"
      # "camera SR"
      # "camera status SR"
      # "histogram SR"
      # "Buffer Index SR"
      n543 = invoke class="Library" method="Release"(reference=w931) -> (reference out=w932:refnum<k24>)  [unwired: 2 in, 2 out]
      n544 = Close Reference(reference=w932) -> ()  [unwired: 1 in, 1 out]
    }
    frame #3 {
      # "We must call GC::Collect() to remove all the references. This is a known issue.\nhttp://www.ni.com/product-documentation/53586/en/#468139_by_Category"
      n545 = invoke class="GC" method="Collect"() -> ()  [unwired: 3 in, 3 out]
    }
  }
  n546 = control-ref of="Color (Off/On)"() -> (w3:refnum<vi>)
  n547 = property class="Bool (strict)"(reference=w3, "Value"=FALSE) -> ()  [unwired: 1 in, 2 out]
  n548 = local write "Image saving path"("Define path in Disk streaming" ("SavingPath")) -> ()
  n549 = local write "Histogram On/Off"(w7) -> ()
  n550 = global write "PVCamGlobalVariables.vi" "Histogram Enabled"(w7) -> ()
  n551 = property on="Exposure" class="DigNum (strict)"("Visible"=w11) -> ()  [unwired: 2 in, 2 out]
  n552 = property on="YBinning" class="DigNum (strict)"("Visible"=w11) -> ()  [unwired: 2 in, 2 out]
  n553 = property on="Y Binning" class="DigNum (strict)"("Visible"=w11) -> ()  [unwired: 2 in, 2 out]
  n554 = property on="X Binning" class="DigNum (strict)"("Visible"=w11) -> ()  [unwired: 2 in, 2 out]
  n555 = property on="CC Max" class="DigNum (strict)"("Visible"=w11) -> ()  [unwired: 2 in, 2 out]
  n556 = property on="Full CCD Y" class="DigNum (strict)"("Visible"=w11) -> ()  [unwired: 2 in, 2 out]
  n557 = property on="Clearing modes" class="DigNum (strict)"("Visible"=w11) -> ()  [unwired: 2 in, 2 out]
  n558 = property on="CC Min" class="DigNum (strict)"("Visible"=w11) -> ()  [unwired: 2 in, 2 out]
  n559 = property on="Full CCD Height" class="DigNum (strict)"("Visible"=w11) -> ()  [unwired: 2 in, 2 out]
  n560 = property on="Exp. out" class="DigNum (strict)"("Visible"=w11) -> ()  [unwired: 2 in, 2 out]
  n561 = property on="XBinning" class="DigNum (strict)"("Visible"=w11) -> ()  [unwired: 2 in, 2 out]
  n562 = property on="Full CCD X" class="DigNum (strict)"("Visible"=w11) -> ()  [unwired: 2 in, 2 out]
  n563 = property on="Full CCD Width" class="DigNum (strict)"("Visible"=w11) -> ()  [unwired: 2 in, 2 out]
  n564 = property on="Trigger Mode" class="DigNum (strict)"("Visible"=w11) -> ()  [unwired: 2 in, 2 out]
  "LabVIEW app version" <- "1.2.1"
  "8 Bit Histogram" <- i32[] [] ("8 Bit Histogram")
  "Capturing" <- FALSE ("Capturing")
  "Buffer Index" <- 0.0 ("Buffer Index")
  "Disk queue size" <- 0.0 ("Queue size")
  "Name" <- "" ("Name")
